vi "Text control 2 v6.6.vi"() -> ()   [LabVIEW 2016]
panel:
  in  "Tab Control":enum32{"Main", "Other parameters"}(tab)
  in  "Plot sample extrema vs time":bool
  out "Line running":i32
  out "Total lines":i32
  out "Path":path=path "C:/users/rlp38/09Apr2009LTtesting/test2.txt"
  out "I vs Vg":cluster{"Y data in":dbl[], "X data in":dbl[]}[](graph)
  out "Is max":dbl format="%.2e"
  out "Id max":dbl format="%.2e"
  out "Ig max":dbl format="%.2e"
  out "Imax vs time":cluster{"Y data in":dbl[], "X data in":dbl[]}[](graph)
  out "Imin vs time":cluster{"Y data in":dbl[], "X data in":dbl[]}[](graph)
  out "I vs Vd":cluster{"Y data in":dbl[], "X data in":dbl[]}[](graph)
  in  "Script":string="#pulsedstressV d 0.03 20 0 0.5 0.0827 5\n#\n#itime m\n#gaterangemode a\n#drainrangemode a\n#pulsed on 0.05 0 0.02\n#transfer d -10 40 1 5 40 35\n#transfer d -10 40 1 5 40 35\n#transfer d -10 40 1 5 40 35\n#output d 0 40 20 0 40 1\n#\n#\n#sample 1 0.008 221 6 0.003\n#samplei 400e-6 200 6 0.002 0.1\n#vsu2pulse -10 4\n#\n#stressV 0.016 0.03 2e-4 0.1e-3 11\n#stressI 220e-7 0.08 15\n#transfer s -1 1 0.5 -0.005 0.005 0.005\n#output s 0 0 0 -0.008 0.008 0.002"
  out "Command running:":string
  out "Serial port data":string
  out "Elapsed Time":dbl caption="Elapsed Time (s)"
  in  "Time Units":u16(ring)=1 items=["Seconds", "Minutes", "Hours"]
  in  "Time Offset":dbl caption="Set Start Time (s)"
  in  "Reset":bool
  in  "Auto Reset":bool
  in  "integration time":u32(slide) max=2 step=1 scale=0.0..2.0
  out "Is on":dbl format="%.2e"
  out "Id on":dbl format="%.2e"
  out "Ig on":dbl format="%.2e"
  out "Ion vs time":cluster{"Y data in":dbl[], "X data in":dbl[]}[](graph)
  out "Ioff vs time":cluster{"Y data in":dbl[], "X data in":dbl[]}[](graph)
  out "Ig min":dbl format="%.2e"
  out "Id min":dbl format="%.2e"
  out "Is min":dbl format="%.2e"
  out "Is off":dbl format="%.2e"
  out "Id off":dbl format="%.2e"
  out "Ig off":dbl format="%.2e"
  in  "Integration time (long)":dbl=0.32 min=0.04 max=2.0 step=0.02 format="%.2f"
  in  "Integration time (short)":dbl=0.0019 min=8e-05 max=0.0019 step=8e-05 format="%^.0e"
  in  "Drain: Compliance":dbl=0.001 format="%.8f"
  in  "Gate: Compliance":dbl=0.001 format="%.8f"
  in  "Interrupt scan":bool
  in  "Interrupt program":bool
  in  "Plot output curve extrema vs time":bool
  in  "Plot transfer curve extrema vs time":bool
  out "I vs time (Bias Stress)":cluster{"Y data in":dbl[], "X data in":dbl[]}[](graph)
  in  "Gate Range\nmode":u16(ring) items=["Auto", "Limited", "Fixed"]
  in  "Gate Range":u8(slide)=6 max=11 scale=0.0..11.0
  in  "Source/Drain\nRange mode":u16(ring) items=["Auto", "Limited", "Fixed"]
  in  "Source/Drain Range":u8(slide)=6 max=11 scale=0.0..11.0
  in  "Panel Controls":T1={"Emergency Stop"=refnum, "TransGraph Max"=1e-05, "Text/Graph (text=false)"=TRUE} {"TransGraph Max" format="%.2e"}
  in  "Panel Controls 2":T2={"Emergency Stop"=refnum, "TransGraph Max"=1e-05, "Text/Graph (text=false)"=TRUE, "TransGraph Min"=1e-11} {"TransGraph Min" format="%.2e"; "TransGraph Max" format="%.2e"}
  out "error out":errorcluster
  in  "Delay before read (ms)":u32=1000
  in  "byte count":u32=64
  in  "Serial End Mode for Reads":u16(ring)=2 items=["None", "LastBit", "TermChar"]
  in  "Timeout (ms)":u32=10000
  in  "Enable Termination\nChar (T)":bool=TRUE
  in  "Termination char\n(0xA = '\\n' = LF)\n(0xD = '\\r' = CR)":u8=13 format="%.0x"
  in  "flow control":u16(ring) items=["None"=0, "XON/XOFF"=1, "RTS/CTS"=2, "DTR/DSR"=4]
  in  "stop bits":u16(ring)=10 items=["1.0"=10, "1.5"=15, "2.0"=20]
  in  "parity":u16(ring) items=["None", "Odd", "Even", "Mark", "Space"]
  in  "data bits":u16=8 min=5 max=8 step=1
  in  "VISA resource name":refnum<visa-resource-name>="COM6"
  in  "baud rate":u32=9600
  out "Timings Indicator":T3
  in  "Timings (overwritten by the Front Panel)":T4={"integration time"=0, "Short/Long integration time"=0.00064, "hold time (sec)"=0.0, "delay time (sec)"=0.0, "Step Time (0 disables)"=0.0, "sweep method"=0, "Pulse period"=0.005, "Base voltage"=0.0, "Pulse width"=0.0005} {"Pulse width" min=0.0005 max=0.1 step=0.0001 format="%.4f"; "Base voltage" format="%^.4e"; "Pulse period" min=0.005 max=1.0 step=0.0001 format="%.4f"; "sweep method" items=["Continuous", "Pulsed"]; "Step Time (0 disables)" format="%.2f"; "delay time (sec)" format="%.4f"; "hold time (sec)" format="%.4f"; "Short/Long integration time" format="%^.0e"; "integration time" scale=0.0..2.0}
  in  "SMU4":cluster{"on/off":bool, "Voltage":dbl} {"Voltage" min=-100.0 max=100.0 format="%.2f"}
  in  "Full Reset":bool
  in  "Standby":T5
  out "SMU4 Indicator":cluster{"on/off":bool, "Voltage":dbl} {"Voltage" min=-100.0 max=100.0 format="%.2f"}
  in  "Gate":T6={"Gate Start"=0.0, "Gate Stop"=2.0, "Gate Step (linear only)"=1.0, "Gate Compliance"=0.0001, "Gate PComp"=0.0, "Range mode"=0, "Range"=6} {"Range" max=11 scale=0.0..11.0; "Range mode" items=["Auto", "Limited", "Fixed"]; "Gate PComp" format="%^.2e"; "Gate Compliance" format="%^.2e"; "Gate Step (linear only)" format="%^.4e"; "Gate Stop" format="%^.4e"; "Gate Start" format="%^.4e"}
  in  "Drain 2":T7={"Drain Start"=0.0, "Drain Stop"=2.0, "Drain Compliance"=0.0001, "Drain Step"=1.0, "Drain PComp"=0.0, "Range mode"=0, "Range"=6} {"Range" max=11 scale=0.0..11.0; "Range mode" items=["Auto", "Limited", "Fixed"]; "Drain PComp" format="%^.2e"; "Drain Step" format="%^.4e"; "Drain Compliance" format="%^.2e"; "Drain Stop" format="%^.4e"; "Drain Start" format="%^.4e"}
  # "Time"
  # "Syntax:\nitime [s|m|l] time(sec): [s|m|l] determines the integration time setting (small|medium|long) and time sets the value.\nNOTE: The value of the integration time has to be within the range allowed by its category (s|m|l), otherwise, the closest value will be used. (e.g. if the category is set to short but the time value is very long, the actual value used will be the maximum short integration time.\nIntegration times:\n    Short: Default: 640 us. Range: 8E-5 - 1.92E-3 seconds.\n    Medium: Fixed at 1 NPL cycle (0.02 seconds).\n    Long: Default: 16 NPL cycles (0.32 seconds). Range: 2-100 NPL cycles (0.04 seconds - 2 seconds).\ngaterangemode [a|l|f]\ndrainrangemode [a|l|f]\npulsed [on|off] PulsePeriod(sec) PulseBaseVoltage PulseONWidth(sec)\nstandby [on l off]\nwait NumMilliseconds\nwait-min NumMinutes\n# texthere = comment\nSMU4 [ON|OFF] Voltage\ntransfer [s|d] VgStart VgStop VgStep VdStart VdStop VdStep\noutput [s|d] VgStart VgStop VgStep VdStart VdStop VdStep\nsample Vg Vd NumSamples Time(s) SampleInterval(s)\nsamplei Idg NumSamples Time(s) SampleInterval(s) VDGcompliance\n100 samples is approximately 13 seconds with medium integration\n# if in doubt use SampleInterval(s) = 0.004\n    NOTE: When doing bias stress measurements, set the Time Units to \"Seconds\", as the \"sample\" command has been configured to give the output to seconds.\nstressV VG VD IGcompliance IDcompliance Duration(sec)\nstressI IDG VDGcompliance Duration(sec)\nvsu2pulse Bias Duration(s)\npulsedstressV [s|d] VEstop VgON VgOFF Period(s) PulseONwidth(s) Vd\nsample-fpp Vg Vd NumSamples Time\nresample-fpp Vg Vd\ntransfer-fpp [s|d] VgStart VgStop VgStep VdStart VdStop VdStep\noutput-fpp [s|d] VgStart VgStop VgStep VdStart VdStop VdStep\nserial SerialPortCommand"
  # "1\n2\n3\n4\n5\n6\n7\n8\n9\n10\n11\n12\n13\n14\n15\n16\n17\n18\n19\n20"
  # "Serial port settings"
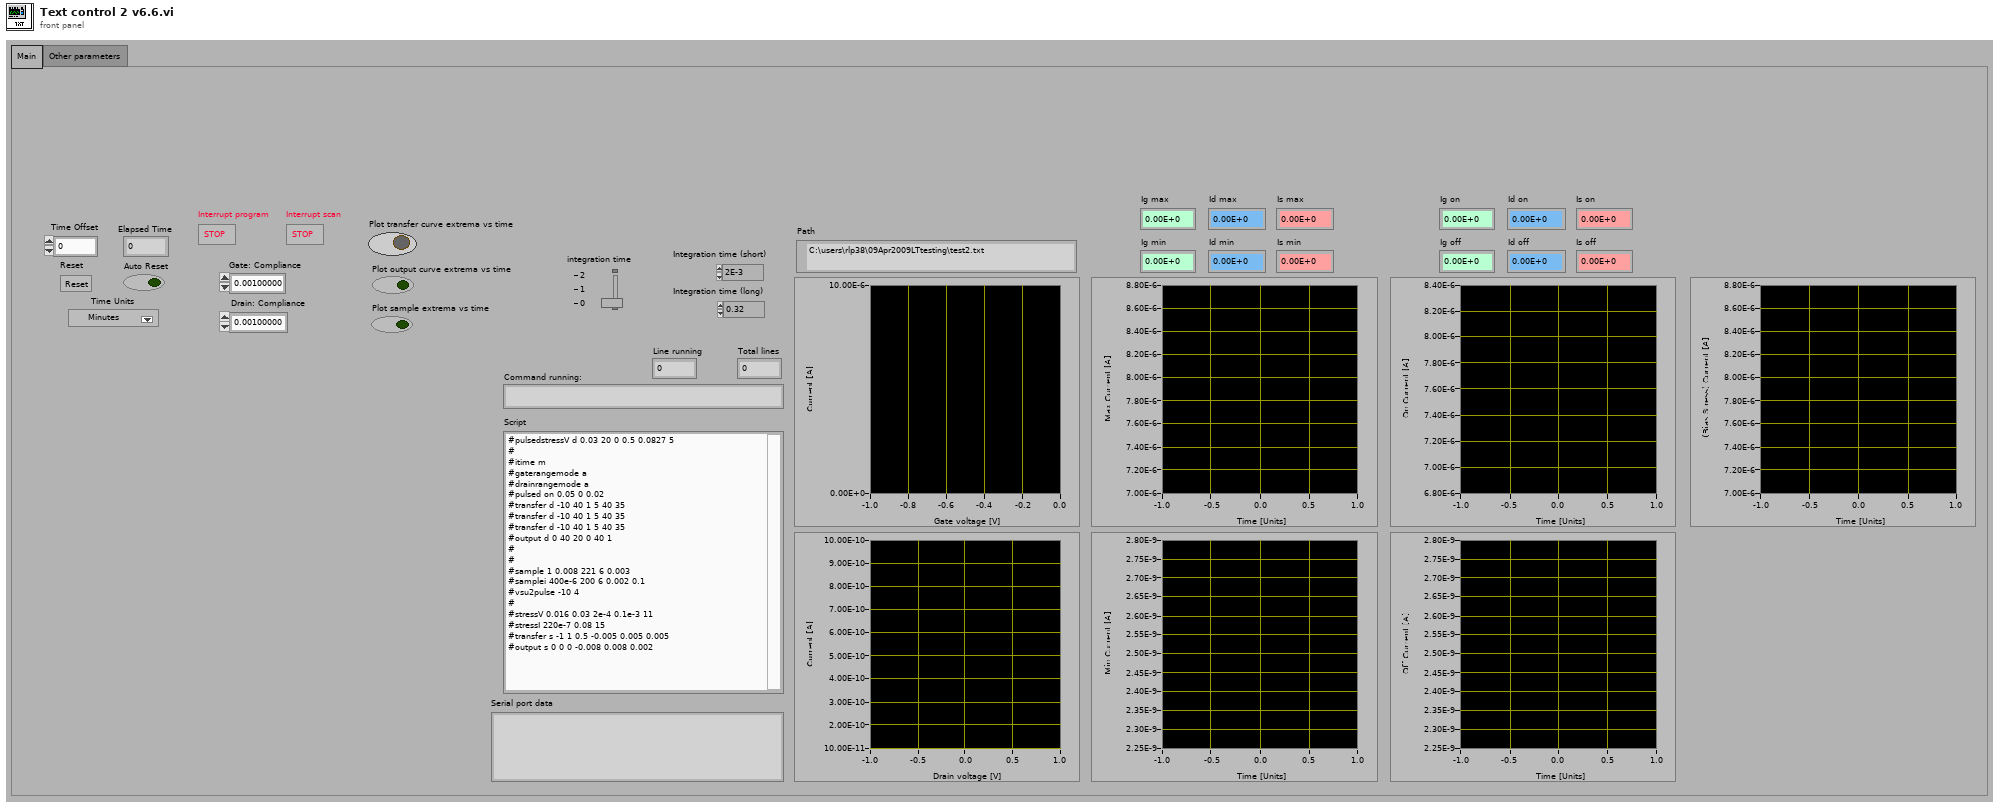
[diagram p1: front panel]
types:
  T1 = cluster{"Emergency Stop":refnum<vi>, "TransGraph Max":dbl, "Text/Graph (text=false)":bool}
  T2 = cluster{"Emergency Stop":refnum<vi>, "TransGraph Max":dbl, "Text/Graph (text=false)":bool, "TransGraph Min":dbl}
  T3 = cluster{"integration time (0:s, 1:m, 2:l)":u32, "Short/Long integration time":dbl, "hold time (sec)":dbl, "delay time (sec)":dbl, "Step Time (0 disables)":dbl, "sweep method":u16, "Pulse period":dbl, "Base voltage":dbl, "Pulse width":dbl}
  T4 = cluster{"integration time":u32, "Short/Long integration time":dbl, "hold time (sec)":dbl, "delay time (sec)":dbl, "Step Time (0 disables)":dbl, "sweep method":u16, "Pulse period":dbl, "Base voltage":dbl, "Pulse width":dbl}
  T5 = cluster{"Gate Standby":bool, "Drain Standby":bool}
  T6 = cluster{"Gate Start":dbl, "Gate Stop":dbl, "Gate Step (linear only)":dbl, "Gate Compliance":dbl, "Gate PComp":dbl, "Range mode":u16, "Range":u8}
  T7 = cluster{"Drain Start":dbl, "Drain Stop":dbl, "Drain Compliance":dbl, "Drain Step":dbl, "Drain PComp":dbl, "Range mode":u16, "Range":u8}
  T8 = enum16{"open", "replace", "create", "open or create", "replace or create", "replace or create with confirmation"}
  T9 = cluster{"V2 Start":dbl, "V2 Step":dbl, "Number of points":i32}
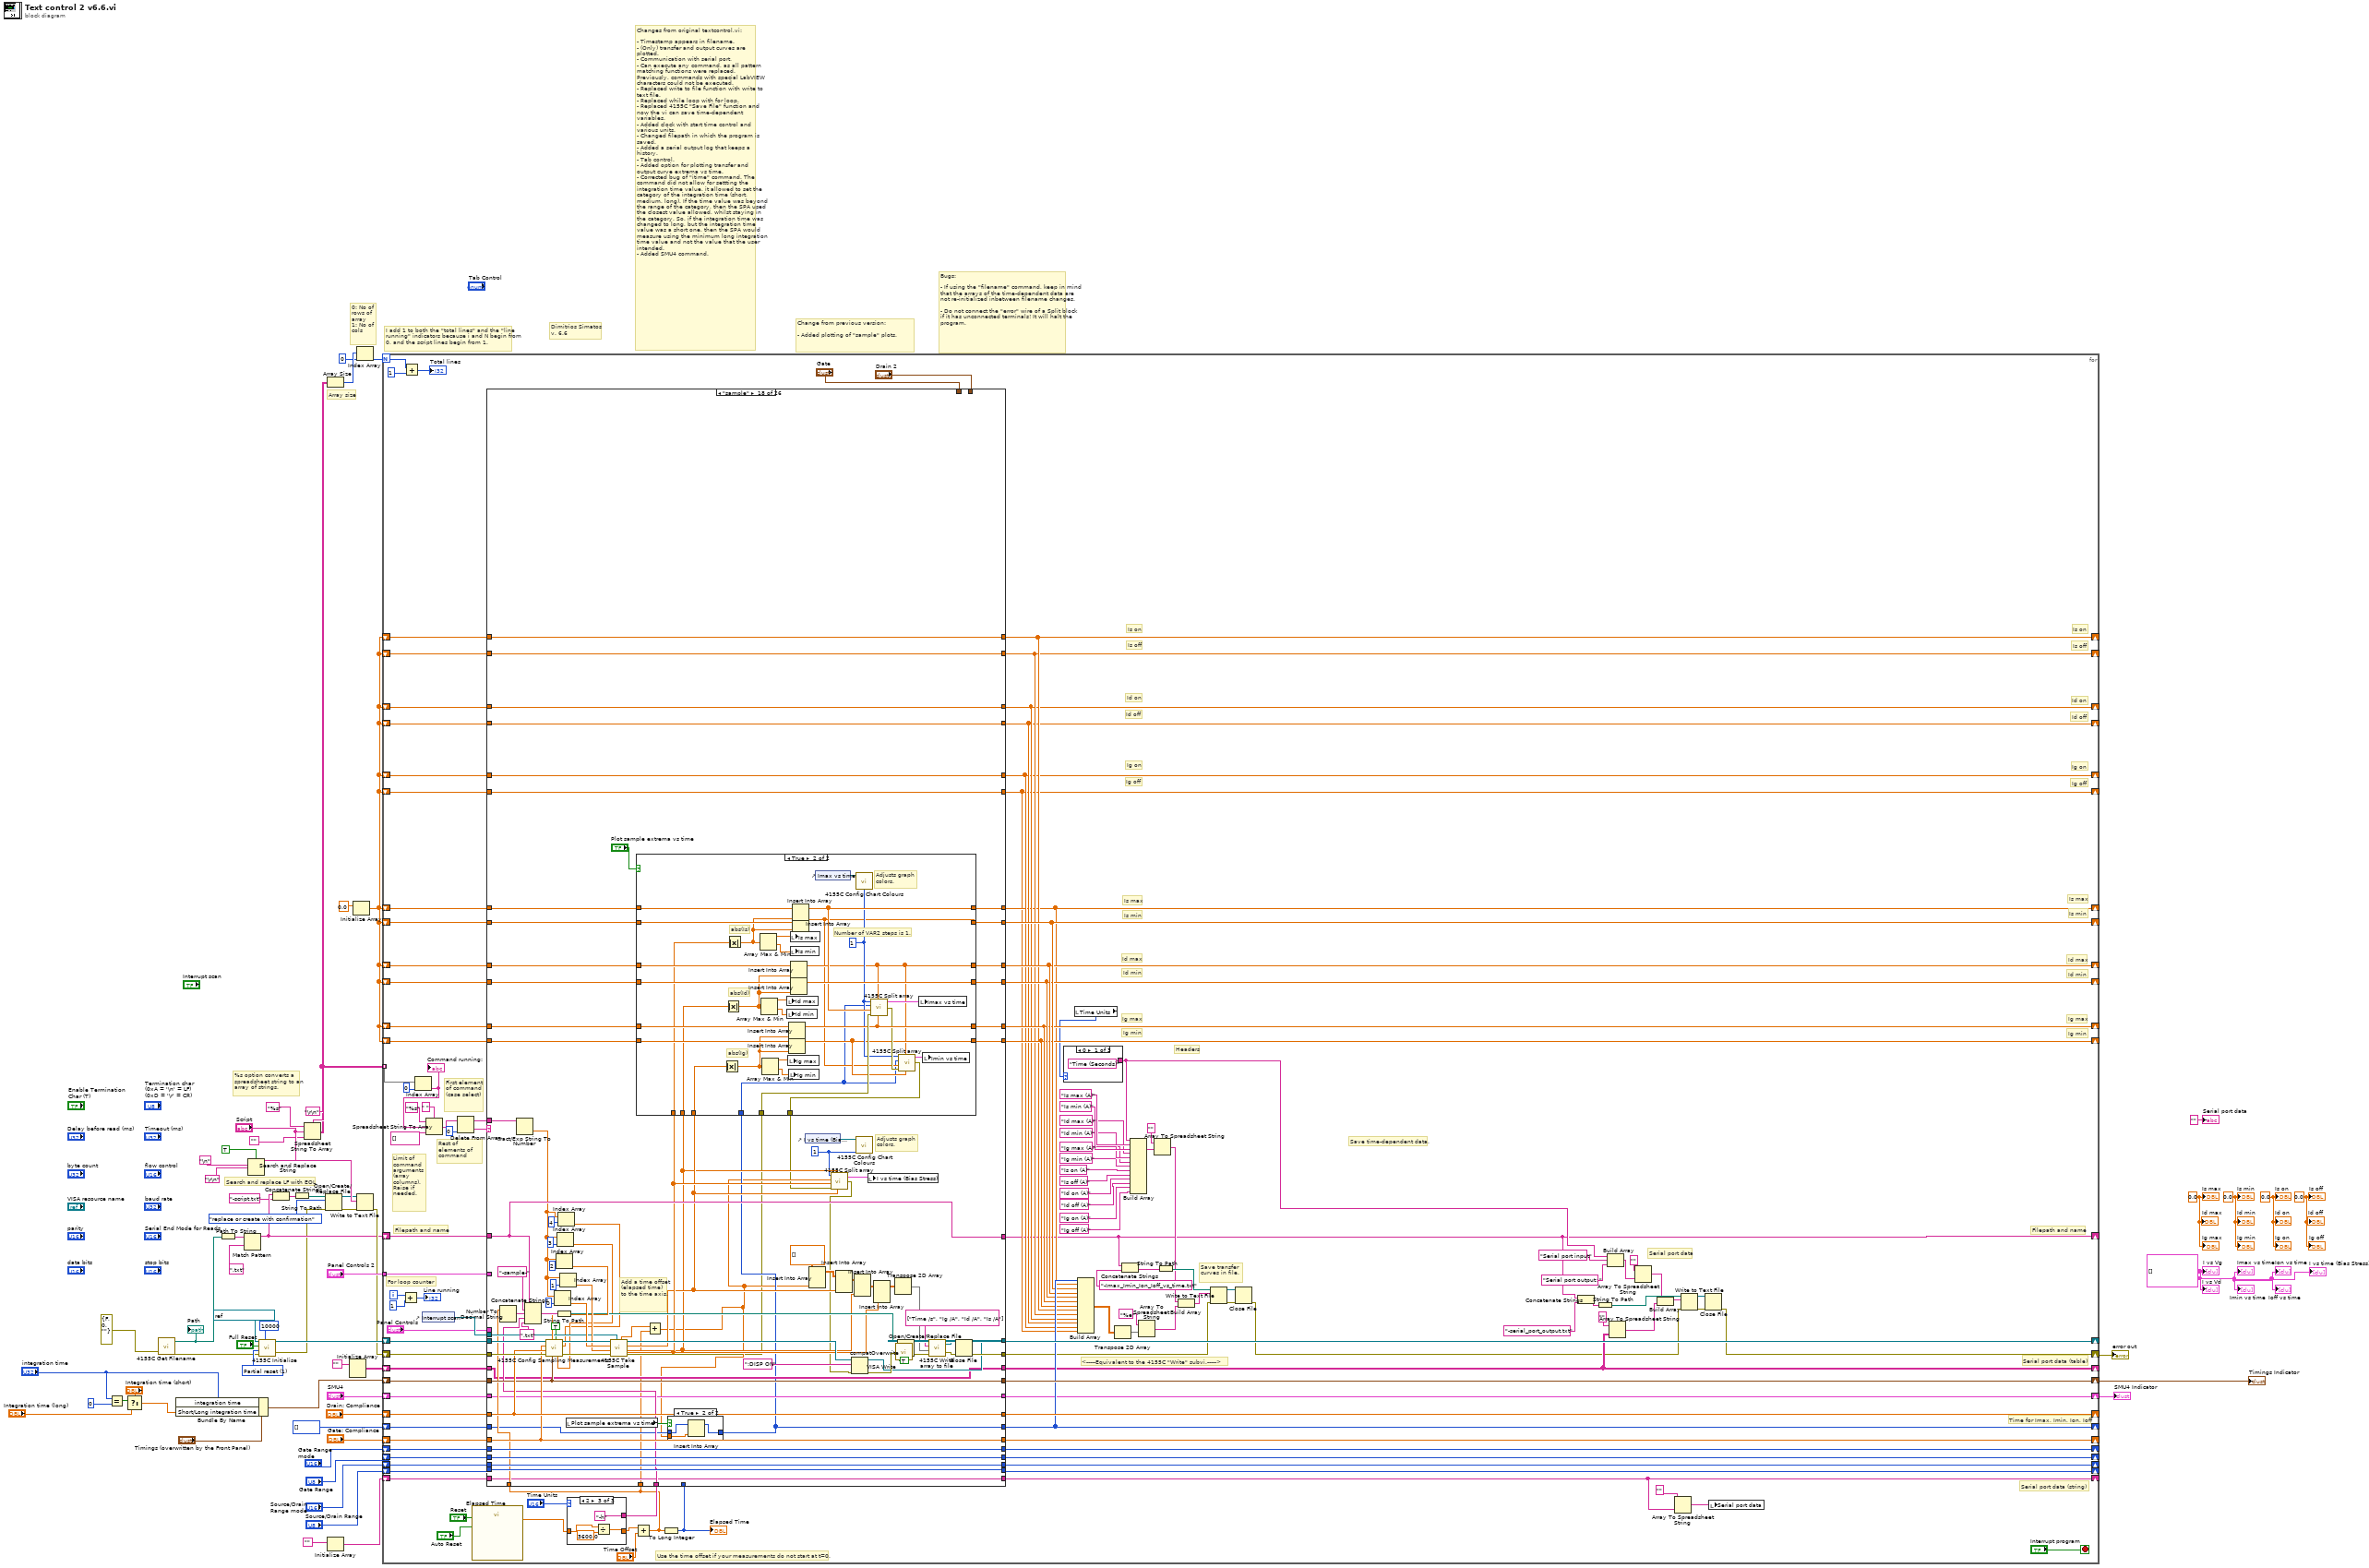
[diagram p0: block diagram]
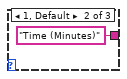
[diagram p2: hidden frame]
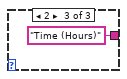
[diagram p3: hidden frame]
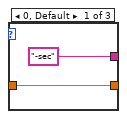
[diagram p4: hidden frame]
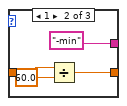
[diagram p5: hidden frame]
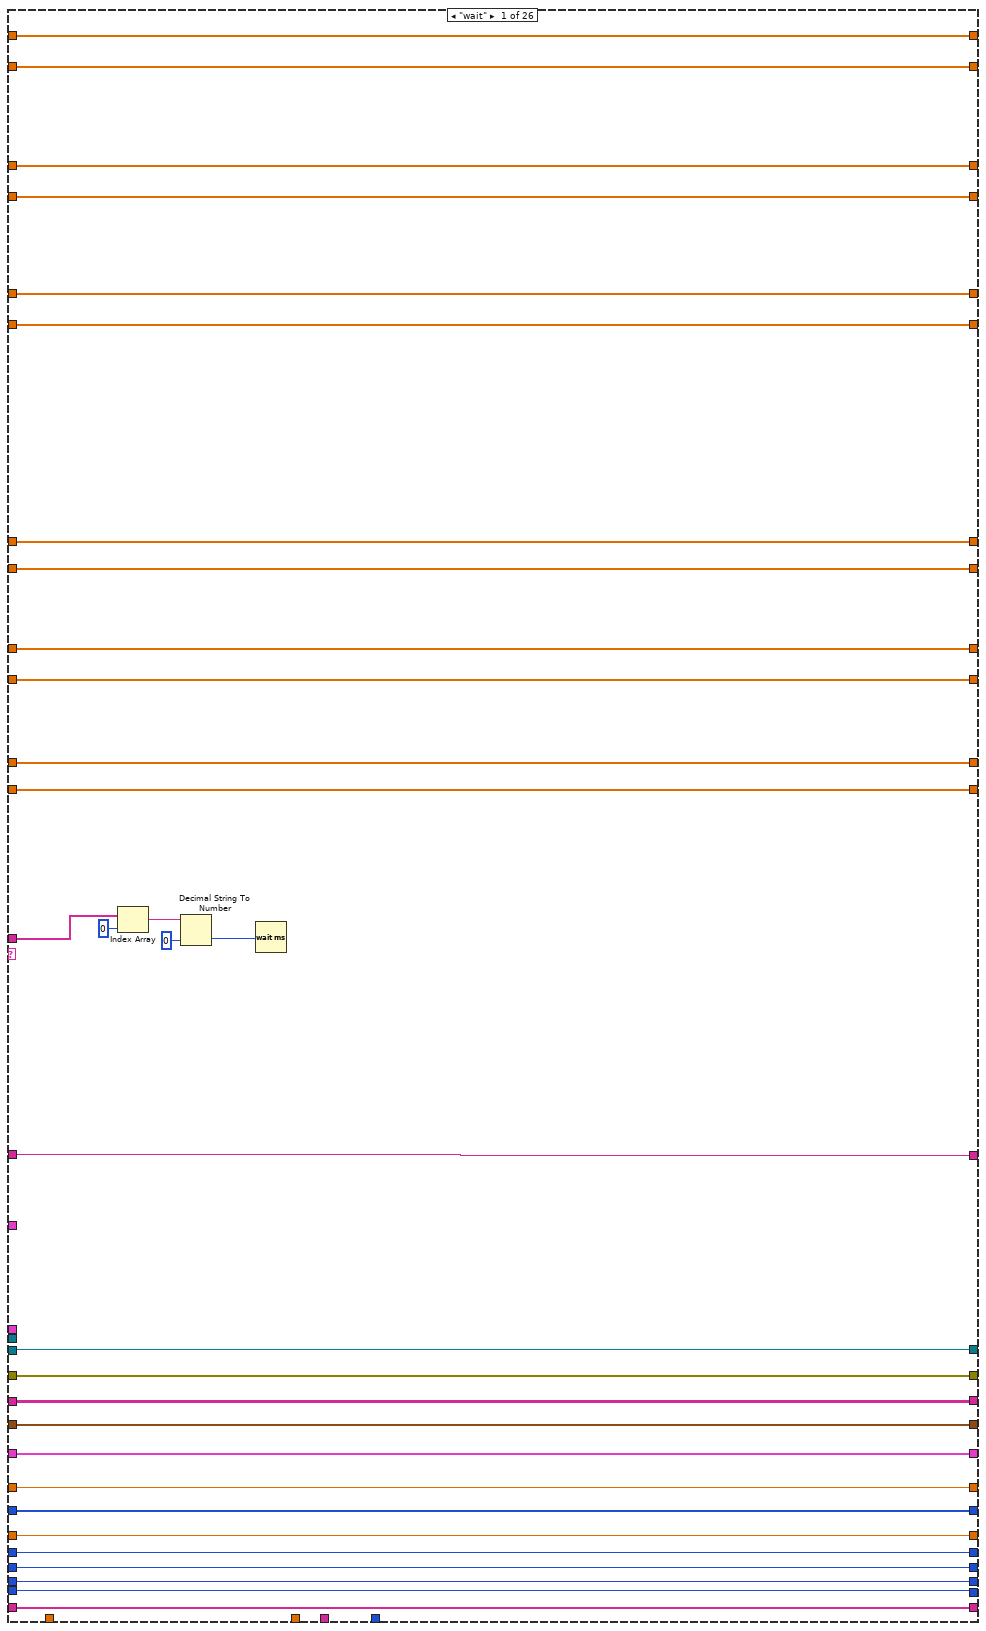
[diagram p6: hidden frame]
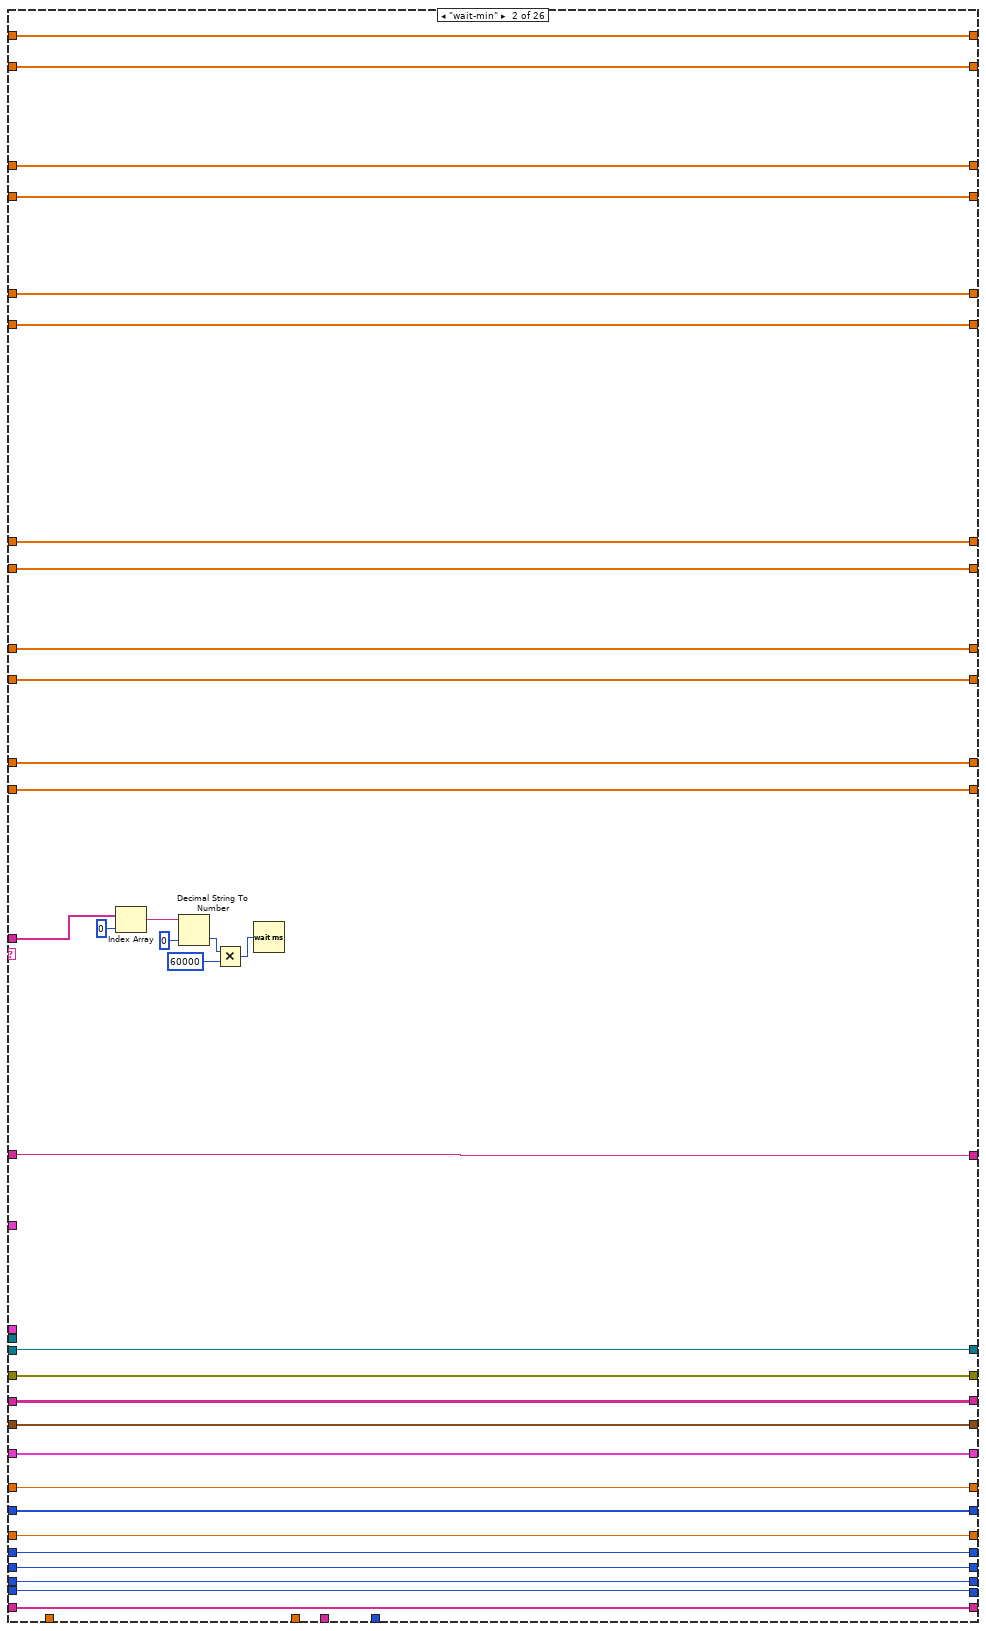
[diagram p7: hidden frame]
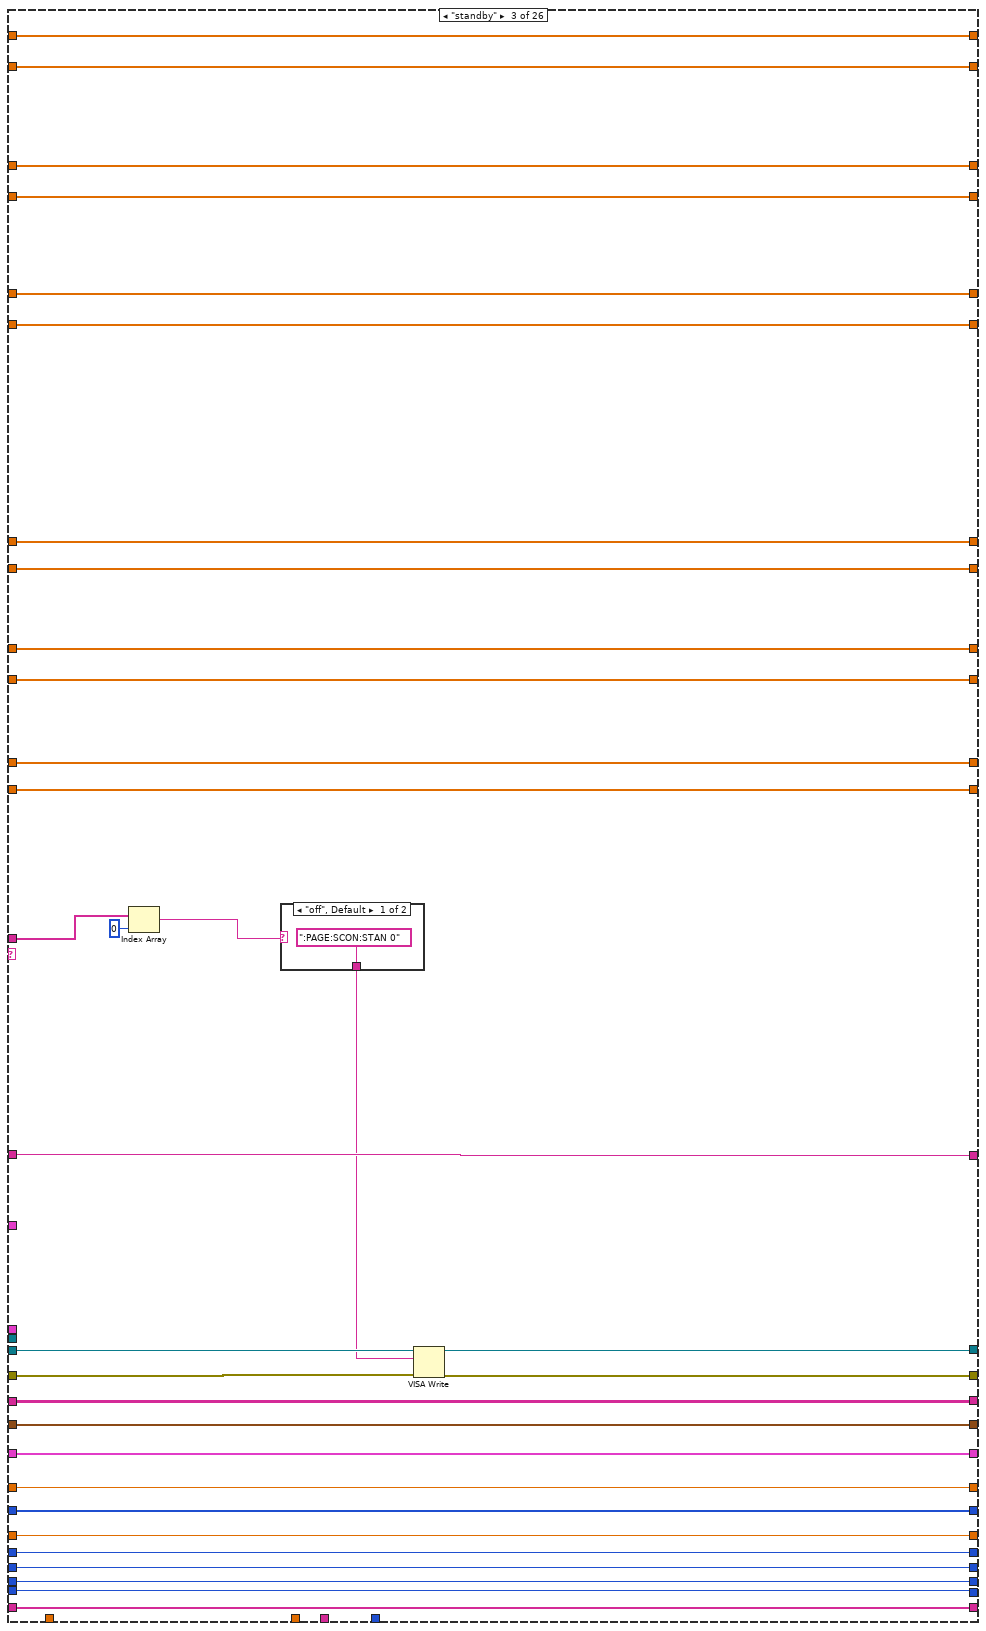
[diagram p8: hidden frame]
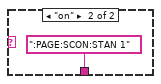
[diagram p9: hidden frame]
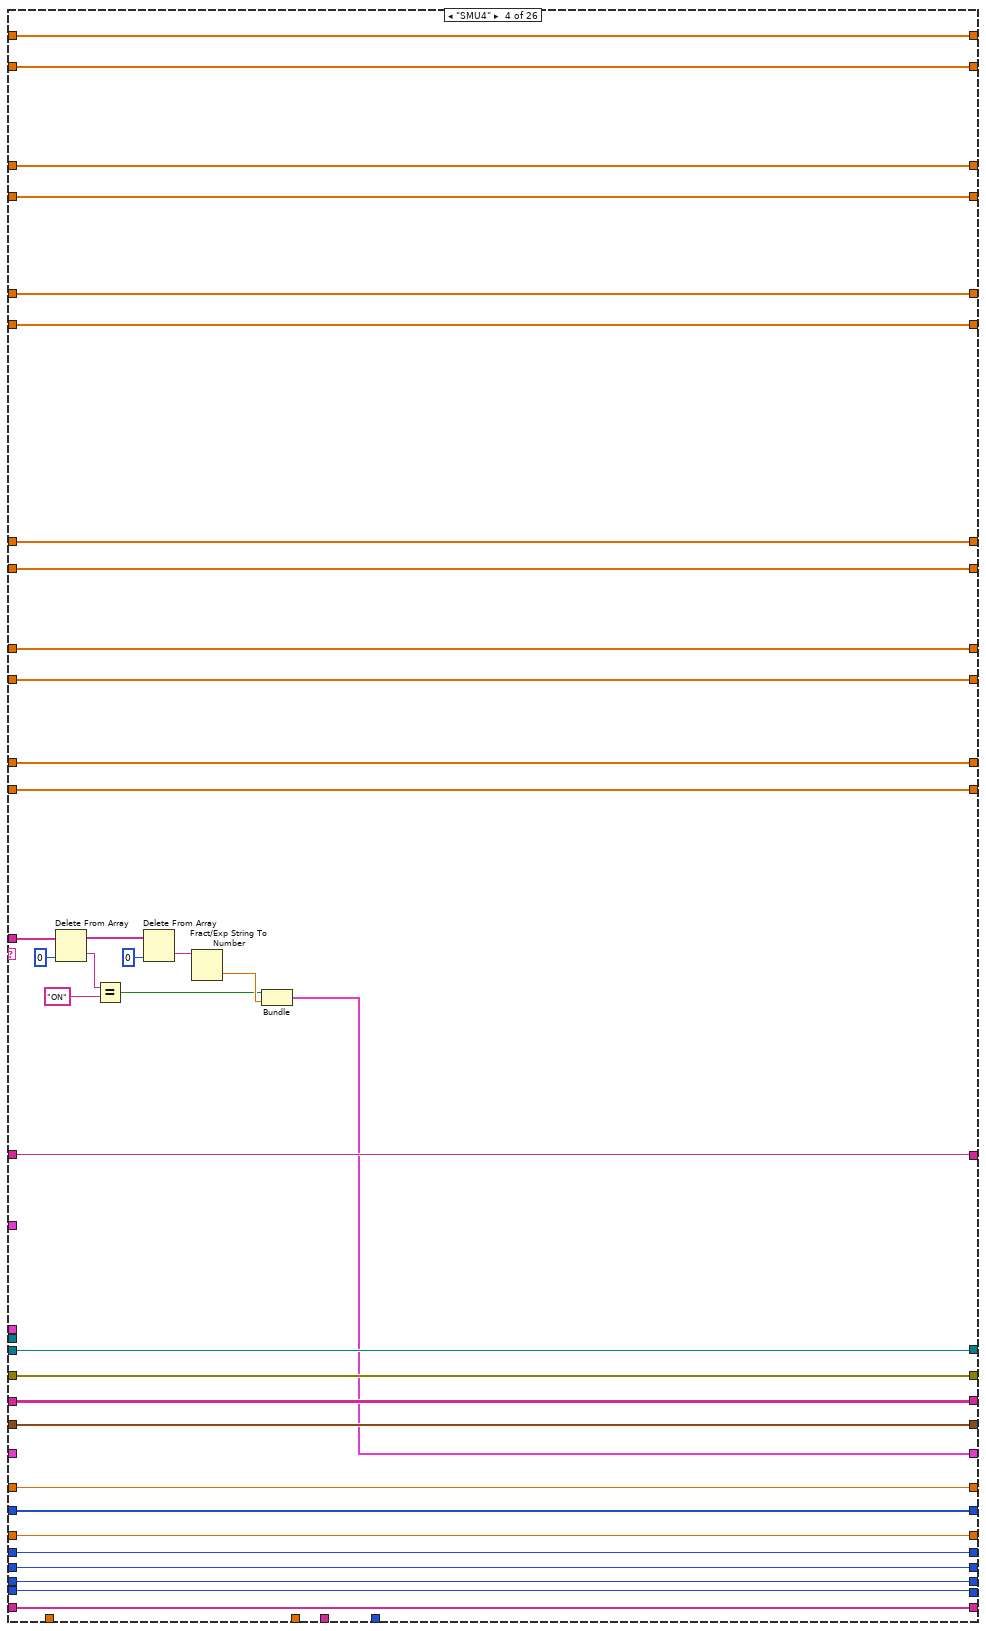
[diagram p10: hidden frame]
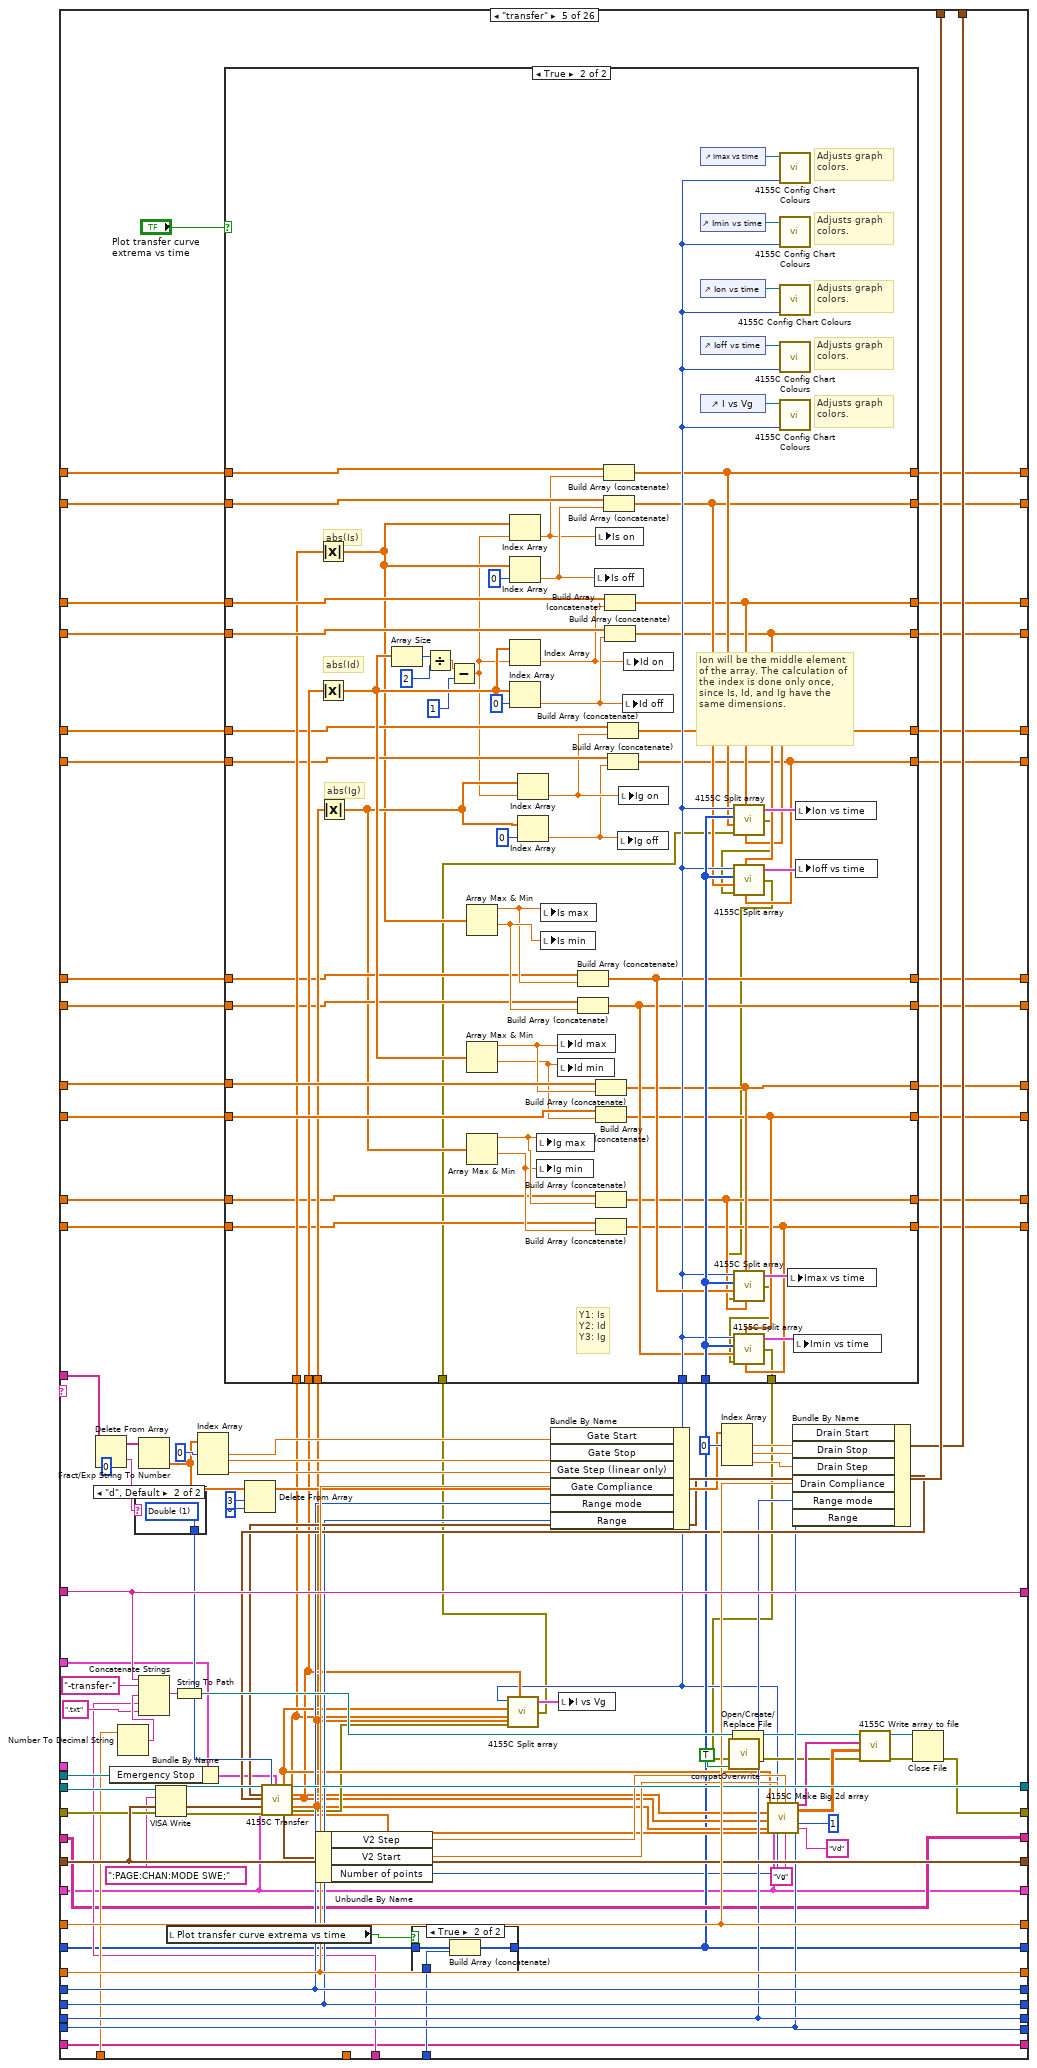
[diagram p11: hidden frame]
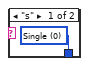
[diagram p14: hidden frame]
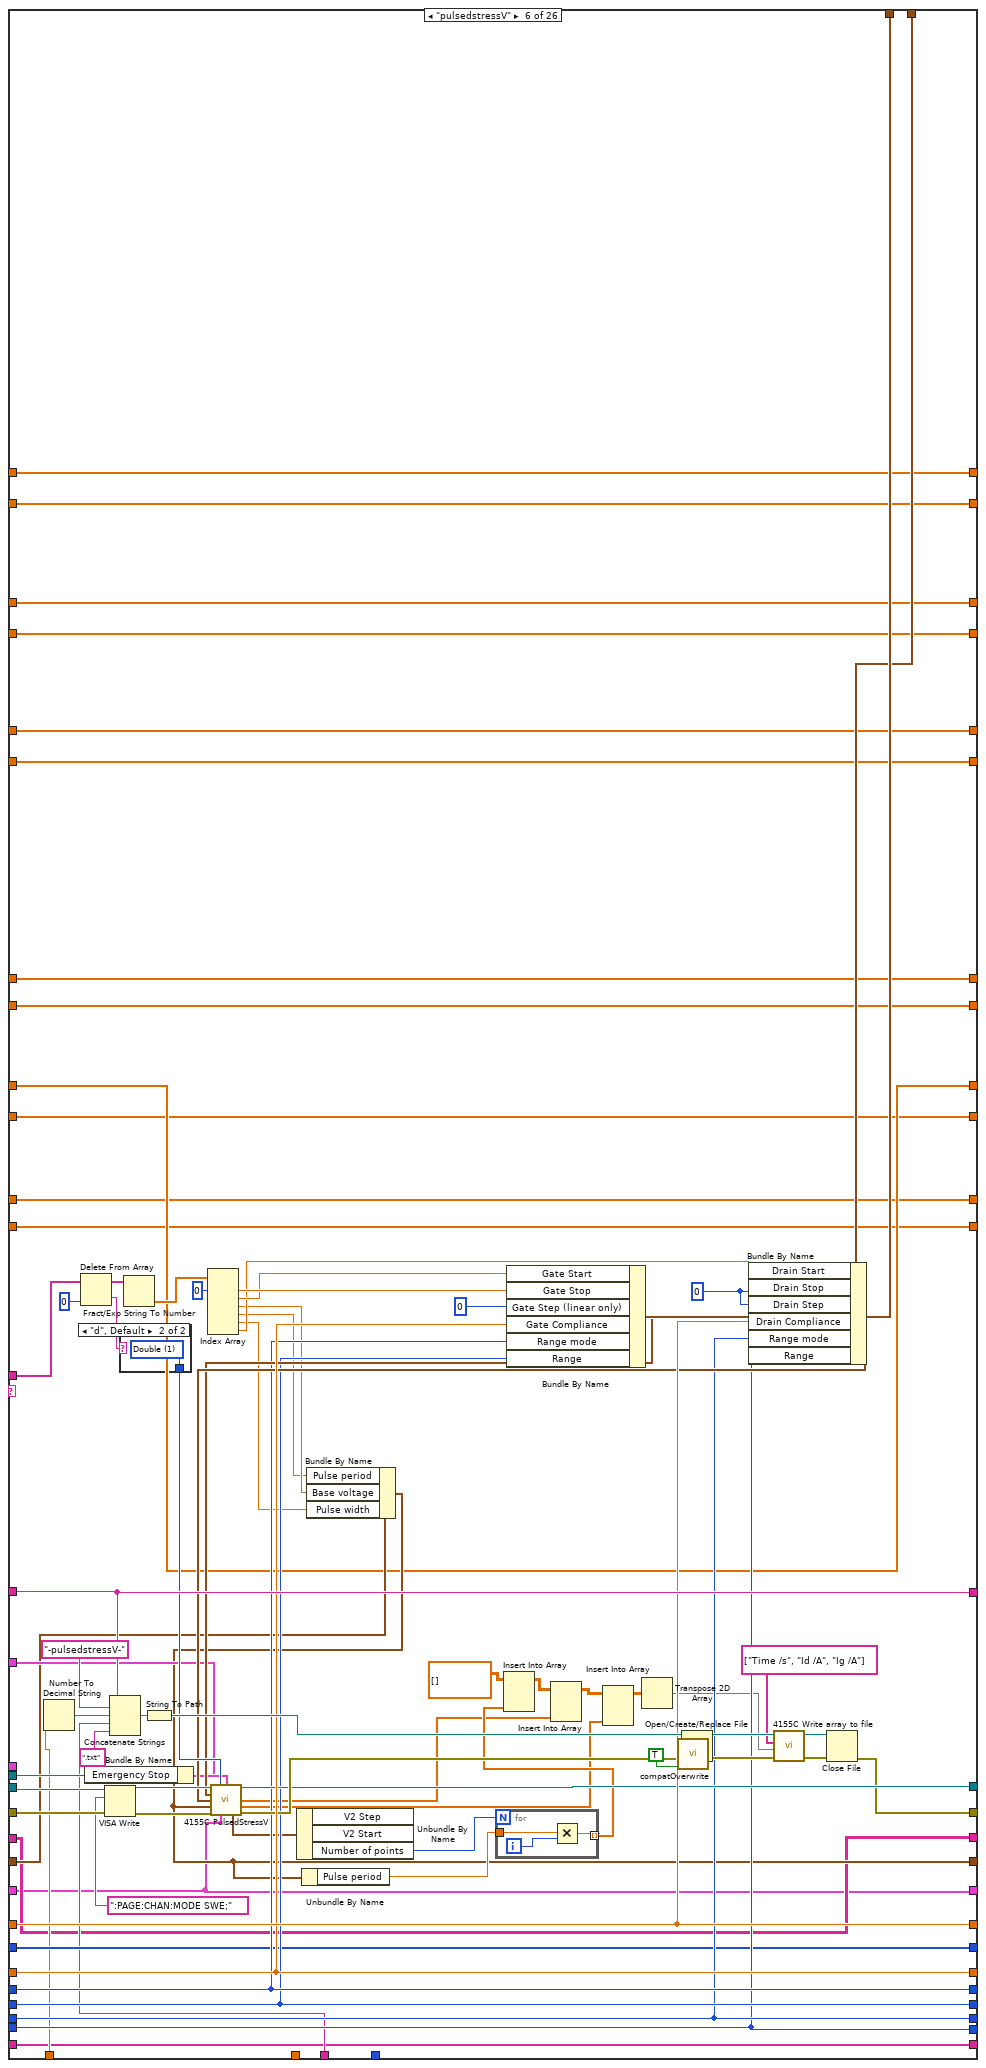
[diagram p15: hidden frame]
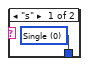
[diagram p16: hidden frame]
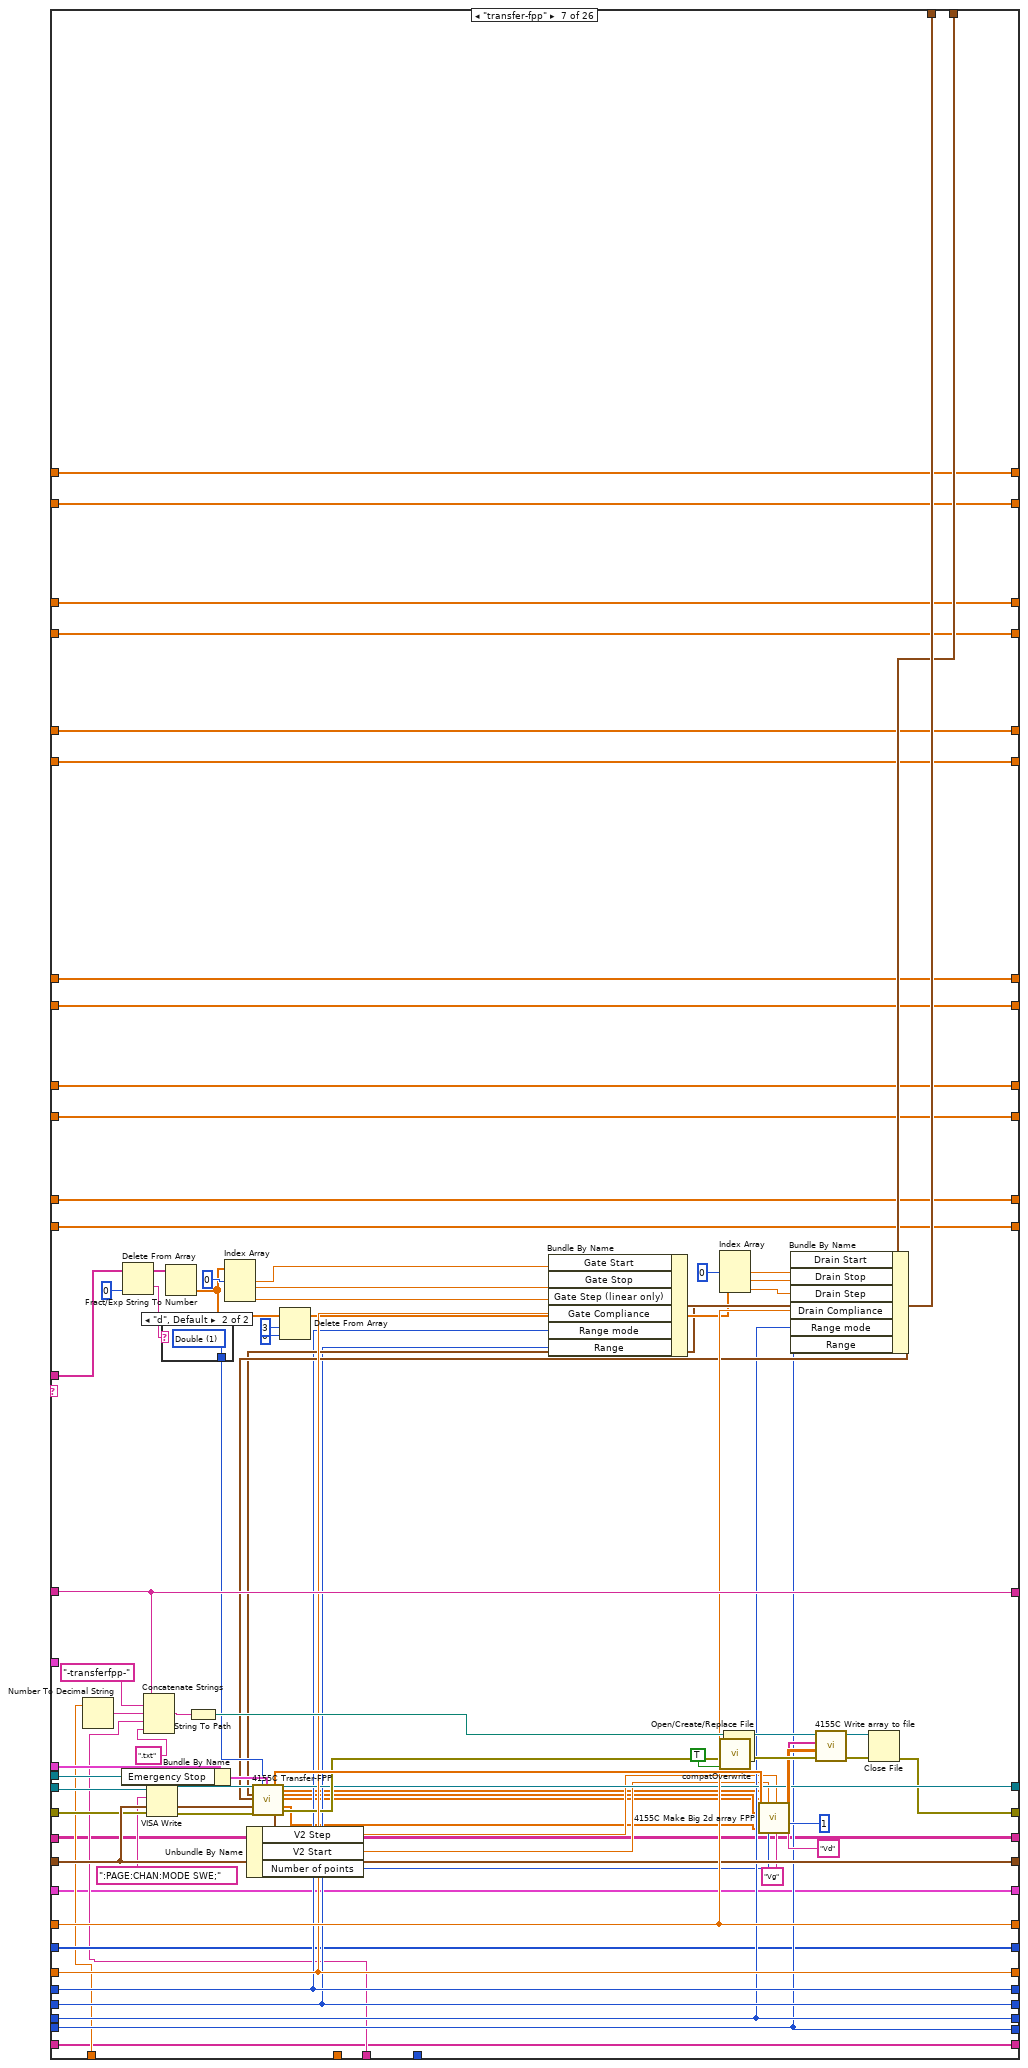
[diagram p17: hidden frame]
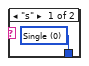
[diagram p18: hidden frame]
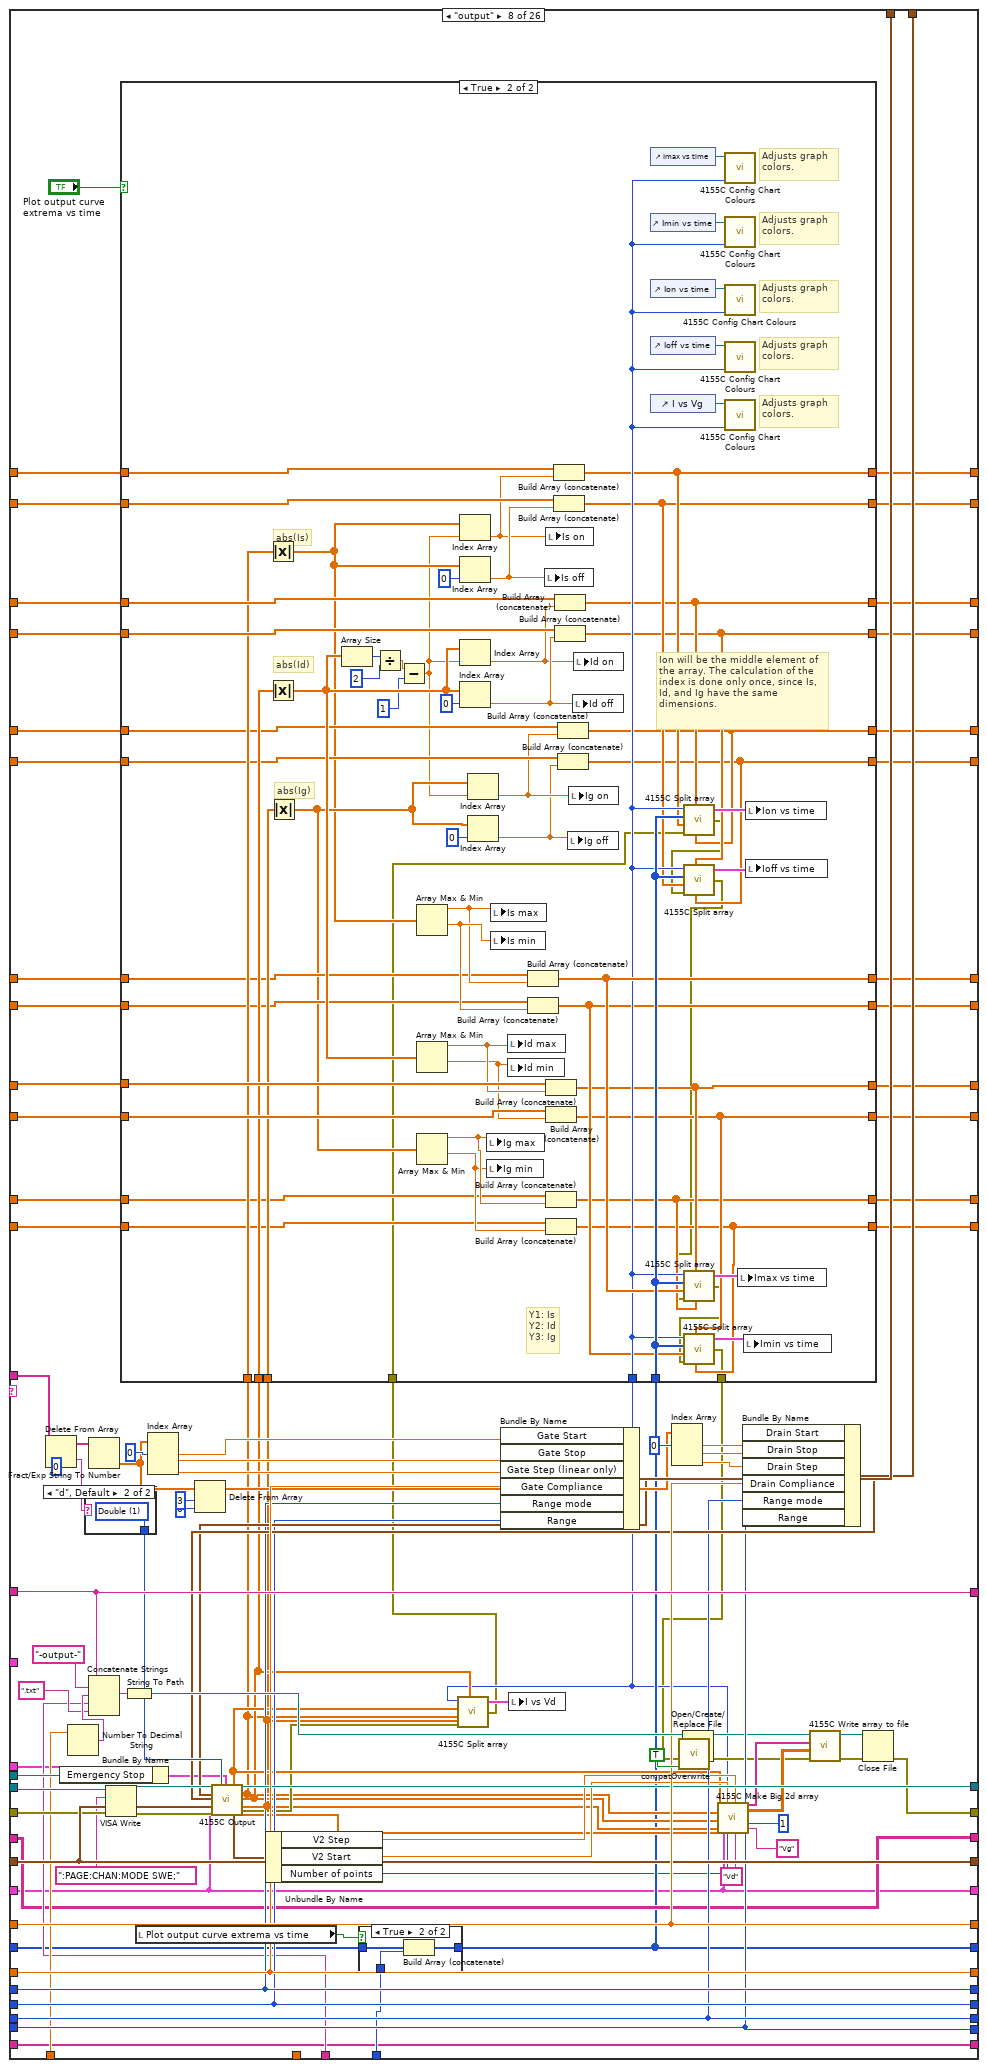
[diagram p19: hidden frame]
diagram:
  w1 = cluster{"Y data in":dbl[], "X data in":dbl[]}[] [] ("I vs Vg")
  w9 = 0.0 ("Is off")
  w10 = 0.0 ("Is on")
  w11 = 0.0 ("Is min")
  w12 = 0.0 ("Is max")
  w58 = u16 1 items=["Reset All", "Partial reset"] ("Type of reset")
  # "Change from previous version:\n\n- Added plotting of \"sample\" plots."
  # "I add 1 to both the \"total lines\" and the \"line running\" indicators because i and N begin from 0, and the script lines begin from 1."
  # "Bugs:\n\n- If using the \"filename\" command, keep in mind that the arrays of the time-dependent data are not re-initialized inbetween filename changes. \n\n- Do not connect the \"error\" wire of a Split block if it has unconnected terminals! It will halt the program."
  # "Array size"
  # "%s option converts a spreadsheet string to an array of strings."
  # "0: No of rows of array\n1: No of cols"
  # "Dimitrios Simatos\nv. 6.6"
  # "Changes from original textcontrol.vi:\n\n- Timestamp appears in filename.\n- (Only) transfer and output curves are plotted.\n- Communication with serial port.\n- Can execute any command, as all pattern matching functions were replaced. Previously, commands with special LabVIEW characters could not be executed.\n- Replaced write to file function with write to text file.\n- Replaced while loop with for loop.\n- Replaced 4155C \"Save File\" function and now the vi can save time-dependent variables.\n- Added clock with start time control and various units.\n- Changed filepath in which the program is saved.\n- Added a serial output log that keeps a history.\n- Tab control.\n- Added option for plotting transfer and output curve extrema vs time.\n- Corrected bug of \"itime\" command. The command did not allow for settting the integration time value, it allowed to set the category of the integration time (short, medium, long). If the time value was beyond the range of the category, then the SPA used the closest value allowed, whilst staying in the category. So, if the integration time was changed to long, but the integration time value was a short one, then the SPA would measure using the minimum long integration time value and not the value that the user intended.\n- Added SMU4 command."
  # "Search and replace LF with EOL"
  n1 = Equal?(x="integration time", y=u32 0) -> (x = y?=w59:bool)
  n2 = Select(t="Integration time (short)", s=w59, f="Integration time (long)") -> (s? t:f=w17:dbl)
  n3 = call "4155C Get Filename.vi"("error in (no error)"=errorcluster {"status"=FALSE, "code"=0, "source"=""}) -> ("error out"=w53:errorcluster, "path"=w28:path)  [unwired: 2 in, 1 out]
  "Path" <- w28
  n4 = Bundle By Name(cluster="Timings (overwritten by the Front Panel)", "integration time"="integration time", "Short/Long integration time"=w17) -> (w51:T4)
  n5 = Path To String(path=w28) -> (string=w29:string)
  n6 = Match Pattern(string=w29, regular expression=".txt") -> (before substring=w15:string)  [unwired: 1 in, 3 out]
  n7 = Search and Replace String(replace all?=TRUE ("replace all? (F)"), input string="Script", search string="\n", replace string="\r\n") -> (result string=w41:string)  [unwired: 4 in, 3 out]
  n8 = call "4155C Initialise.vi"("VISA resource name in"=refnum<visa-resource-name> "GPIB0::14::INSTR", "Reset"="Full Reset", "Type of reset"=w58, "error in (no error)"=w53, "VISA Timeout Value"=u32 10000) -> ("VISA Resource Name out"=w52:refnum<visa-resource-name>, "error out"=w7:errorcluster)
  n9 = Concatenate Strings(w15, "-script.txt" ("string")) -> (w16:string)
  n10 = String To Path(string=w16) -> (path=w5:path)
  n11 = Spreadsheet String To Array(delimiter (Tab)="\r\n", format string="%s", spreadsheet string="Script", array type (2D Dbl)="") -> (array=w32:string[][])
  n12 = Open/Create/Replace File(file path (use dialog)=w5, error in=w7, operation (0:open)=T8."replace or create with confirmation") -> (refnum out=w4:refnum<file>, error out=w6:errorcluster)  [unwired: 3 in, 1 out]
  n13 = Array Size(array=w32) -> (size(s)=w36:i32[])
  n14 = Initialize Array("") -> (w21:string[])  [unwired: 1 in]
  n15 = Initialize Array("") -> (w19:string[][])  [unwired: 2 in]
  n16 = Initialize Array(0.0 ("element")) -> (w23:dbl[])  [unwired: 1 in]
  n17 = Index Array(array=w36, index=0) -> (element=w34:i32)
  n18 = Write to Text File(file (use dialog)=w4, text=w41, error in=w6) -> (error out=w25:errorcluster)  [unwired: 1 in, 2 out]
  n19 = for {
    N: w34 -> [w133]
    shift-left: "Source/Drain Range" -> [w173]
    shift-right: [w169] -> _
    shift-left: "Source/Drain\nRange mode" -> [w174]
    shift-right: [w170] -> _
    shift-left: "Gate Range" -> [w175]
    shift-right: [w171] -> _
    shift-left: "Gate Range\nmode" -> [w176]
    shift-right: [w172] -> _
    shift-left: "Gate: Compliance" -> [w185]
    shift-right: [w181] -> _
    shift-left: "Drain: Compliance" -> [w186]
    shift-right: [w182] -> _
    shift-left: w51 -> [w187]
    shift-right: [w183] -> w18
    shift-left: w25 -> [w188]
    shift-right: [w70] -> w27
    shift-left: w52 -> [w189]
    shift-right: [w184] -> _
    shift-left: w15 -> [w190]
    shift-right: [w73] -> _
    tunnel: "Panel Controls 2" -> [w167]
    shift-right: [w85] -> _
    shift-left: w23 -> [w166]
    shift-right: [w120] -> _
    shift-left: i32[] [] -> [w162]
    tunnel: w32 -> [w161] mode=indexing
    shift-right: [w84] -> _
    shift-left: w23 -> [w138]
    shift-right: [w115] -> _
    shift-left: w21 -> [w125]
    shift-right: [w116] -> _
    shift-left: w19 -> [w118]
    shift-right: [w78] -> _
    shift-left: w23 -> [w106]
    shift-right: [w79] -> _
    shift-left: w23 -> [w105]
    shift-right: [w83] -> _
    shift-left: w23 -> [w94]
    shift-right: [w82] -> _
    shift-left: w23 -> [w93]
    shift-right: [w76] -> _
    shift-left: w23 -> [w92]
    shift-right: [w86] -> _
    shift-left: w23 -> [w91]
    shift-right: [w77] -> _
    shift-left: w23 -> [w90]
    shift-right: [w75] -> _
    shift-left: w23 -> [w89]
    shift-right: [w81] -> _
    shift-left: w23 -> [w88]
    shift-right: [w80] -> _
    shift-left: w23 -> [w87]
    shift-right: [w66] -> w2
    shift-left: "SMU4" -> [w168]
    i -> [w128]
    stop <- "Interrupt program" stop-if-true
    # "Is off"
    # "Is on"
    # "Ig off"
    # "Ig on"
    # "Is min"
    # "Is max"
    # "Ig min"
    # "Ig max"
    # "Id min"
    # "Id max"
    # "Id off"
    # "Id on"
    # "Is off"
    # "Is on"
    # "Ig off"
    # "Ig on"
    # "Is min"
    # "Is max"
    # "Ig min"
    # "Ig max"
    # "Id min"
    # "Id max"
    # "Id off"
    # "Id on"
    # "Filepath and name"
    # "Limit of command arguments (array columns). Raise if needed."
    # "Serial port data (string)"
    # "Serial port data (table)"
    # "Serial port data"
    # "For loop counter"
    # "<-----Equivalent to the 4155C \"Write\" subvi.----->"
    # "Headers"
    # "Save transfer curves in file."
    # "Filepath and name"
    # "Save time-dependent data."
    # "Use the time offset if your measurements do not start at t=0."
    # "Time for Imax, Imin, Ion, Ioff"
    # "Rest of elements of command"
    # "First element of command\n(case select)"
    n20 = Add(x=w128, y=1) -> (x+y=→"Line running":i32)
    n21 = Add(x=w133, y=1) -> (x+y=→"Total lines":i32)
    n22 = Index Array(array=w161, index=0 ("line index")) -> (element=w156:string)
    "Command running:" <- w156
    n23 = control-ref of="Interrupt scan"() -> (w180:refnum<vi>)
    n24 = Spreadsheet String To Array(delimiter (Tab)=" ", format string="%s", spreadsheet string=w156, array type (2D Dbl)=string[] []) -> (array=w154:string[])
    n25 = Delete From Array(array=w154, index=0) -> (deleted portion=w107:string, array with subset deleted=w153:string[])  [unwired: 1 in]
    n26 = call "Elapsed Time"("Reset"="Reset", "Auto Reset"="Auto Reset") -> ("Elapsed Time (s)"=w163:dbl)  [unwired: 10 in, 7 out]
    n27 = case shown="2" "Time Units" {
      tunnel: ["-sec" "-min" "-h"] -> w164
      tunnel: [w194 w198 w201] -> w134
      tunnel: w163 -> [w194 w197 w202]
      frame 0, Default {
      }
      frame 1 {
        n28 = Divide(x=w197, y=60.0) -> (x/y=w198:dbl)
      }
      frame 2 {
        n29 = Divide(x=w202, y=3600.0) -> (x/y=w201:dbl)
      }
    }
    n30 = Add(x=w134, y="Time Offset") -> (x+y=w64:dbl)
    n31 = To Long Integer(number=w64) -> (32bit integer=w65:i32)
    "Elapsed Time" <- w65
    n32 = case shown="\"sample\"" w107 {
      tunnel: w153 -> [w234 w267 w299 w311 w428 w535 w670 w785 w941 w969 w1038 w1079 w1118 w1153 w1181 _ _ w1345 w1461 _ w1554 w1612 w1668 w1752 w1828 w1862]
      tunnel: w190 -> [w229 w263 w297 w324 w435 w594 w678 w792 w949 w986 w1027 w1071 w1111 w1147 w1174 w1207 w1263 w1326 w1443 w1488 w1541 w1599 w1656 w1746 w1824 w1864]
      tunnel: w189 -> [w228 w262 w288 w323 w406 w579 w647 w763 w917 w987 w1028 w1072 w1112 w1148 w1175 w1212 w1265 w1351 w1467 w1492 w1560 w1618 w1674 w1758 w1782 w1868]
      tunnel: w188 -> [w227 w261 w287 w322 w405 w578 w646 w762 w914 w988 w1029 w1073 w1113 w1149 w1176 w1211 w1236 w1350 w1466 w1491 w1559 w1617 w1673 w1757 w1781 w1867]
      tunnel: w187 -> [w226 w260 w296 w320 w431 w555 w674 w788 w945 w996 w1037 w1070 w1110 w1146 w1173 w1210 w1260 w1318 w1435 w1497 w1534 w1592 w1649 w1745 w1823 w1869]
      tunnel: w186 -> [w225 w259 w295 w319 w433 w592 w676 w790 w947 w995 w1036 w1078 w1117 w1152 w1180 w1209 w1245 w1349 w1465 w1500 w1558 w1616 w1672 w1756 w1832 w1870]
      tunnel: w185 -> [w224 w258 w294 w317 w432 w591 w675 w789 w946 w994 w1035 w1077 w1116 w1151 w1179 w1208 w1246 w1327 w1444 w1499 w1542 w1600 w1657 w1747 w1825 w1872]
      tunnel: [w228 w262 w286 w323 w430 w589 w672 w787 w943 w987 w1028 w1072 w1112 w1148 w1175 w1212 w1265 w1319 w1417 w1490 w1535 w1593 w1650 w1698 w1784 w1868] -> w184
      tunnel: [w227 w261 w285 w322 w429 w588 w671 w786 w942 w988 w1029 w1073 w1113 w1149 w1176 w1211 w1235 w1328 w1418 w1489 w1543 w1601 w1658 w1697 w1783 w1866] -> w119
      tunnel: [w226 w260 w296 w320 w431 w551 w674 w788 w945 w989 w1030 w1070 w1110 w1146 w1173 w1210 w1260 w1318 w1435 w1497 w1534 w1592 w1649 w1745 w1823 w1869] -> w183
      tunnel: [w225 w259 w295 w319 w433 w592 w676 w790 w947 w995 w1036 w1078 w1117 w1152 w1180 w1209 w1245 w1349 w1465 w1500 w1558 w1616 w1672 w1756 w1832 w1870] -> w182
      tunnel: [w224 w258 w294 w317 w432 w591 w675 w789 w946 w994 w1035 w1077 w1116 w1151 w1179 w1208 w1246 w1327 w1444 w1499 w1542 w1600 w1657 w1747 w1825 w1872] -> w181
      tunnel: [w229 w263 w297 w324 w435 w594 w678 w792 w949 w986 w1027 w1071 w1111 w1147 w1174 w1207 w1263 w1326 w1443 w1488 w1541 w1599 w1656 w1746 w1824 w1864] -> w73
      tunnel: w180 -> [_ _ _ _ w437 w598 w683 w794 w953 _ _ _ _ _ _ _ _ w1323 w1440 _ w1540 w1598 w1655 w1718 w1800 _]
      tunnel: "Gate" -> [_ _ _ _ w415 w582 w657 w772 w928 _ _ _ _ _ _ _ _ _ _ _ _ _ _ _ _ _]
      tunnel: "Drain 2" -> [_ _ _ _ w414 w581 w656 w771 w927 _ _ _ _ _ _ _ _ _ _ _ _ _ _ _ _ _]
      tunnel: "Panel Controls" -> [_ _ _ _ _ _ w655 w698 w926 _ _ _ _ _ _ _ _ _ _ _ _ _ _ _ _ _]
      tunnel: w176 -> [w223 w257 w293 w316 w399 w572 w640 w756 w912 w993 w1034 _ w1109 w1145 w1172 w1206 w1247 w1314 w1431 w1493 w1530 w1588 w1645 w1741 w1819 w1873]
      tunnel: w175 -> [w222 w256 w292 w315 w398 w571 w639 w755 w911 w992 w1033 w1076 _ w1136 w1178 w1205 w1248 w1315 w1432 w1494 w1531 w1589 w1646 w1742 w1820 w1874]
      tunnel: w174 -> [w221 w255 w291 w314 w397 w570 w638 w754 w910 w991 w1032 w1075 w1115 w1150 _ w1204 w1249 w1316 w1433 w1495 w1532 w1590 w1647 w1743 w1821 w1875]
      tunnel: w173 -> [w220 w254 w290 w313 w396 w569 w637 w753 w913 w990 w1031 w1074 w1114 _ w1177 w1203 w1250 w1317 w1434 w1496 w1533 w1591 w1648 w1744 w1822 w1876]
      tunnel: [w223 w257 w293 w316 w399 w572 w640 w756 w912 w993 w1034 w1069 w1109 w1145 w1172 w1206 w1247 w1314 w1431 w1493 w1530 w1588 w1645 w1741 w1819 w1873] -> w172
      tunnel: [w222 w256 w292 w315 w398 w571 w639 w755 w911 w992 w1033 w1076 w1101 w1136 w1178 w1205 w1248 w1315 w1432 w1494 w1531 w1589 w1646 w1742 w1820 w1874] -> w171
      tunnel: [w221 w255 w291 w314 w397 w570 w638 w754 w910 w991 w1032 w1075 w1115 w1150 w1171 w1204 w1249 w1316 w1433 w1495 w1532 w1590 w1647 w1743 w1821 w1875] -> w170
      tunnel: [w220 w254 w290 w313 w396 w569 w637 w753 w913 w990 w1031 w1074 w1114 w1137 w1177 w1203 w1250 w1317 w1434 w1496 w1533 w1591 w1648 w1744 w1822 w1876] -> w169
      tunnel: w168 -> [w204 w235 w268 _ w337 w524 w609 w694 w881 w966 w1010 w1053 w1085 w1120 w1155 w1187 w1213 w1301 w1397 w1472 w1501 w1563 w1621 w1677 w1759 w1833]
      tunnel: w167 -> [_ _ _ _ w390 w566 _ _ _ _ _ _ _ _ _ _ _ _ _ _ _ _ _ _ _ _]
      tunnel: [w219 w250 w283 w328 w352 w543 w627 w710 w899 w985 w1025 w1068 w1100 w1135 w1170 w1202 w1231 w1291 w1401 w1487 w1519 w1581 w1639 w1695 w1777 w1865] -> w85
      tunnel: w166 -> [w219 w250 w283 w328 w387 w543 w627 w745 w899 w985 w1025 w1068 w1100 w1135 w1170 w1202 w1231 w1297 w1401 w1487 w1519 w1581 w1639 w1695 w1777 w1865]
      tunnel: w64 -> [_ _ _ _ w386 w540 w625 w744 w896 _ _ _ _ _ _ _ w1229 w1306 w1413 _ w1516 w1578 w1636 w1692 w1773 _]
      tunnel: w164 -> [_ _ _ _ w383 w539 w623 w741 w895 _ _ _ _ _ _ _ w1227 w1304 w1412 _ w1515 w1577 w1635 w1691 w1774 _]
      tunnel: w65 -> [_ _ _ _ w379 _ _ w737 _ _ _ _ _ _ _ _ _ _ _ _ _ _ _ _ _ _]
      tunnel: [w218 w249 w282 w318 w356 w542 w626 w714 w898 w984 w1024 w1067 w1099 w1134 w1169 w1201 w1230 w1273 w1415 w1486 w1518 w1580 w1638 w1694 w1776 w1871] -> w120
      tunnel: w162 -> [w218 w249 w282 w318 w382 w542 w626 w740 w898 w984 w1024 w1067 w1099 w1134 w1169 w1201 w1230 w1275 w1415 w1486 w1518 w1580 w1638 w1694 w1776 w1871]
      tunnel: [w217 w248 w281 w327 w351 w538 w622 w709 w894 w983 w1023 w1066 w1098 w1133 w1168 w1200 w1226 w1290 w1400 w1485 w1514 w1576 w1634 w1690 w1772 w1860] -> w84
      tunnel: w138 -> [w217 w248 w281 w327 w378 w538 w622 w736 w894 w983 w1023 w1066 w1098 w1133 w1168 w1200 w1226 w1296 w1400 w1485 w1514 w1576 w1634 w1690 w1772 w1860]
      tunnel: [w216 w247 w280 w312 w371 w537 w621 w729 w893 w982 w1022 w1065 w1097 w1132 w1167 w1199 w1225 w1303 w1411 w1484 w1513 w1575 w1633 w1689 w1771 w1859] -> w115
      tunnel: w125 -> [w216 w247 w280 w312 w371 w537 w621 w729 w893 w982 w1022 w1065 w1097 w1132 w1167 w1199 w1225 w1303 w1411 w1484 w1513 w1575 w1633 w1689 w1771 w1858]
      tunnel: [w215 w246 w279 w321 w370 w536 w620 w728 w892 w981 w1021 w1064 w1096 w1131 w1166 w1198 w1224 w1302 w1410 w1483 w1512 w1574 w1632 w1688 w1770 w1844] -> w116
      tunnel: w118 -> [w215 w246 w279 w321 w370 w536 w620 w728 w892 w981 w1021 w1064 w1096 w1131 w1166 w1198 w1224 w1302 w1410 w1483 w1512 w1574 w1632 w1688 w1770 w1844]
      tunnel: [w213 w244 w277 w333 w345 w533 w618 w703 w890 w979 w1020 w1063 w1094 w1129 w1164 w1196 w1222 w1284 w1409 w1482 w1511 w1573 w1630 w1687 w1769 w1843] -> w78
      tunnel: w106 -> [w213 w244 w277 w333 w369 w533 w618 w727 w890 w979 w1020 w1063 w1094 w1129 w1164 w1196 w1222 w1284 w1409 w1482 w1511 w1573 w1630 w1687 w1769 w1843]
      tunnel: [w214 w245 w278 w334 w346 w534 w619 w704 w891 w980 w1019 w1062 w1095 w1130 w1165 w1197 w1223 w1285 w1408 w1481 w1510 w1572 w1631 w1686 w1768 w1842] -> w79
      tunnel: w105 -> [w214 w245 w278 w334 w368 w534 w619 w726 w891 w980 w1019 w1062 w1095 w1130 w1165 w1197 w1223 w1285 w1408 w1481 w1510 w1572 w1631 w1686 w1768 w1842]
      tunnel: [w206 w237 w270 w326 w350 w530 w616 w708 w888 w972 w1017 w1060 w1092 w1127 w1162 w1194 w1215 w1289 w1399 w1480 w1503 w1565 w1623 w1679 w1763 w1835] -> w83
      tunnel: w94 -> [w206 w237 w270 w326 w364 w530 w616 w722 w888 w972 w1017 w1060 w1092 w1127 w1162 w1194 w1215 w1295 w1399 w1480 w1503 w1565 w1623 w1679 w1763 w1835]
      tunnel: [w205 w236 w269 w325 w349 w531 w617 w707 w889 w971 w1018 w1061 w1093 w1128 w1163 w1195 w1214 w1288 w1398 w1479 w1502 w1564 w1622 w1678 w1762 w1834] -> w82
      tunnel: w93 -> [w205 w236 w269 w325 w363 w531 w617 w721 w889 w971 w1018 w1061 w1093 w1128 w1163 w1195 w1214 w1294 w1398 w1479 w1502 w1564 w1622 w1678 w1762 w1834]
      tunnel: [w208 w239 w272 w330 w355 w529 w614 w713 w886 w977 w1015 w1058 w1090 w1125 w1160 w1192 w1217 w1293 w1403 w1474 w1505 w1567 w1625 w1681 w1761 w1839] -> w76
      tunnel: w92 -> [w208 w239 w272 w330 w362 w529 w614 w720 w886 w977 w1015 w1058 w1090 w1125 w1160 w1192 w1217 w1299 w1403 w1474 w1505 w1567 w1625 w1681 w1761 w1839]
      tunnel: [w207 w238 w271 w329 w353 w532 w615 w711 w887 w978 w1016 w1059 w1091 w1126 w1161 w1193 w1216 w1292 w1402 w1473 w1504 w1566 w1624 w1680 w1760 w1838] -> w86
      tunnel: w91 -> [w207 w238 w271 w329 w361 w532 w615 w719 w887 w978 w1016 w1059 w1091 w1126 w1161 w1193 w1216 w1298 w1402 w1473 w1504 w1566 w1624 w1680 w1760 w1838]
      tunnel: [w210 w241 w274 w332 w344 w528 w612 w702 w884 w975 w1013 w1056 w1088 w1123 w1158 w1190 w1219 w1283 w1405 w1476 w1507 w1569 w1627 w1683 w1765 w1841] -> w77
      tunnel: w90 -> [w210 w241 w274 w332 w360 w528 w612 w718 w884 w975 w1013 w1056 w1088 w1123 w1158 w1190 w1219 w1283 w1405 w1476 w1507 w1569 w1627 w1683 w1765 w1841]
      tunnel: [w209 w240 w273 w331 w343 w527 w613 w701 w885 w976 w1014 w1057 w1089 w1124 w1159 w1191 w1218 w1282 w1404 w1475 w1506 w1568 w1626 w1682 w1764 w1840] -> w75
      tunnel: w89 -> [w209 w240 w273 w331 w359 w527 w613 w717 w885 w976 w1014 w1057 w1089 w1124 w1159 w1191 w1218 w1282 w1404 w1475 w1506 w1568 w1626 w1682 w1764 w1840]
      tunnel: [w212 w243 w276 w336 w348 w526 w610 w706 w882 w973 w1011 w1054 w1086 w1121 w1156 w1188 w1221 w1287 w1407 w1478 w1509 w1571 w1629 w1685 w1767 w1837] -> w81
      tunnel: w88 -> [w212 w243 w276 w336 w358 w526 w610 w716 w882 w973 w1011 w1054 w1086 w1121 w1156 w1188 w1221 w1287 w1407 w1478 w1509 w1571 w1629 w1685 w1767 w1837]
      tunnel: [w211 w242 w275 w335 w347 w525 w611 w705 w883 w974 w1012 w1055 w1087 w1122 w1157 w1189 w1220 w1286 w1406 w1477 w1508 w1570 w1628 w1684 w1766 w1836] -> w80
      tunnel: w87 -> [w211 w242 w275 w335 w357 w525 w611 w715 w883 w974 w1012 w1055 w1087 w1122 w1157 w1189 w1220 w1286 w1406 w1477 w1508 w1570 w1628 w1684 w1766 w1836]
      tunnel: [w204 w235 w268 w302 w337 w524 w609 w694 w881 w966 w1010 w1053 w1085 w1120 w1155 w1187 w1213 w1301 w1397 w1472 w1501 w1563 w1621 w1677 w1759 w1833] -> w66
      tunnel: w64 -> [_ _ _ _ _ _ _ _ _ _ _ _ _ _ _ _ _ w1266 _ _ _ _ _ _ _ _]
      frame "wait" {
        n33 = Index Array(array=w234, index=0 ("Index")) -> (element=w232:string)
        n34 = Decimal String To Number(string=w232, default (0L)=u32 0) -> (number=w231:u32)  [unwired: 1 in, 1 out]
        n35 = Wait (ms)(milliseconds to wait=w231) -> ()  [unwired: 1 out]
      }
      frame "wait-min" {
        n36 = Index Array(array=w267, index=0 ("Index")) -> (element=w265:string)
        n37 = Decimal String To Number(string=w265, default (0L)=u32 0) -> (number=w253:u32)  [unwired: 1 in, 1 out]
        n38 = Multiply(x=w253, y=u32 60000) -> (x*y=w252:u32)
        n39 = Wait (ms)(milliseconds to wait=w252) -> ()  [unwired: 1 out]
      }
      frame "standby" {
        n40 = Index Array(array=w299, index=0 ("Index")) -> (element=w289:string)
        n41 = case shown="\"off\", Default" w289 {
          tunnel: [":PAGE:SCON:STAN 0" ":PAGE:SCON:STAN 1"] -> w284
          frame "off", Default {
          }
          frame "on" {
          }
        }
        n42 = VISA Write(VISA resource name=w288, write buffer=w284, error in (no error)=w287) -> (VISA resource name out=w286:refnum<visa-resource-name>, error out=w285:errorcluster)  [unwired: 1 out]
      }
      frame "SMU4" {
        n43 = Delete From Array(array=w311, index=0) -> (deleted portion=w305:string, array with subset deleted=w308:string[])  [unwired: 1 in]
        n44 = Equal?(x=w305, y="ON") -> (x = y?=w303:bool)
        n45 = Delete From Array(array=w308, index=0) -> (deleted portion=w307:string)  [unwired: 1 in, 1 out]
        n46 = Fract/Exp String To Number(string=w307) -> (number=w304:dbl)  [unwired: 3 in, 1 out]
        n47 = Bundle(w303, w304) -> (w302:cluster{bool, dbl})  [unwired: 1 in]
      }
      frame "transfer" {
        n48 = Delete From Array(array=w428, index=0 ("Index")) -> (deleted portion=w426:string, array with subset deleted=w425:string[])  [unwired: 1 in]
        n49 = Bundle By Name(cluster=w390, "Emergency Stop"=w437) -> (w391:T2)
        n50 = Number To Decimal String(number=w386) -> (decimal integer string=w385:string)  [unwired: 1 in]
        n51 = case shown="\"d\", Default" w426 {
          tunnel: [w522 w523] -> w424
          frame "s" {
            w522 = u16 0 items=["Single", "Double"] ("sweep mode")
          }
          frame "d", Default {
            w523 = u16 1 items=["Single", "Double"] ("sweep mode")
          }
        }
        n52 = Fract/Exp String To Number(string=w425) -> (number=w410:dbl[])  [unwired: 3 in, 1 out]
        n53 = Concatenate Strings(w435, "-transfer-" ("Prefix"), w385, w383, ".txt" ("Suffix (transfer)")) -> (w436:string)
        n54 = VISA Write(VISA resource name=w406, write buffer=":PAGE:CHAN:MODE SWE;" ("write buffer (\"\")"), error in (no error)=w405) -> (VISA resource name out=w403:refnum<visa-resource-name>, error out=w404:errorcluster)  [unwired: 1 out]
        n55 = local read "Plot transfer curve extrema vs time"() -> (w338:bool)
        n56 = String To Path(string=w436) -> (path=w434:path)
        n57 = Index Array(array=w410, index #1=0 ("Index")) -> (element #1=w423:dbl, element #2=w422:dbl, element #3=w421:dbl)  [unwired: 2 in]
        n58 = Delete From Array(array=w410, length=3 ("Length"), index=0 ("Index")) -> (array with subset deleted=w408:dbl[])  [unwired: 1 out]
        n59 = case shown="True" w338 {
          tunnel: w382 -> [w439 w442]
          tunnel: w379 -> [_ w441]
          tunnel: [w439 w440] -> w356
          frame False {
          }
          frame True {
            n60 = Build Array (concatenate)(w442, w441) -> (w440:i32[])
          }
        }
        n61 = Bundle By Name(cluster=w415, "Gate Start"=w423, "Gate Stop"=w422, "Gate Step (linear only)"=w421, "Gate Compliance"=w432, "Range mode"=w399, "Range"=w398) -> (w400:T6)
        n62 = Index Array(array=w408, index #1=0 ("Index")) -> (element #1=w418:dbl, element #2=w417:dbl, element #3=w416:dbl)  [unwired: 2 in]
        n63 = call <vilib>:"compatOverwrite.vi"("overwrite (F)"=TRUE) -> ("overwrite?"=w389:T8)
        n64 = Bundle By Name(cluster=w414, "Drain Start"=w418, "Drain Stop"=w417, "Drain Step"=w416, "Drain Compliance"=w433, "Range mode"=w397, "Range"=w396) -> (w401:T7)
        n65 = call "4155C Transfer.vi"("VISA resource name in"=w403, "Gate"=w400, "Drain"=w401, "Timings"=w431, "error in (no error)"=w404, "SMU4"=w337, "sweep mode"=w424, "Panel Controls"=w391) -> ("VG"=w388:dbl[], "Outparams"=w395:T9, "VISA Resource Name out"=w430:refnum<visa-resource-name>, "IS"=w366:dbl[], "ID"=w367:dbl[], "IG"=w365:dbl[], "error out"=w380:errorcluster, "SMU4"=w392:dbl[])  [unwired: 12 in]
        n66 = Unbundle By Name(w395) -> ("V2 Step"=w394:dbl, "V2 Start"=w393:dbl, "Number of points"=w354:i32)
        n67 = call "4155C Split array.vi"("Number of VAR2 steps"=w354, "Y2 data in"=w367, "X data in"=w388, "Y1 data in"=w366, "Y3 data in"=w365, "error in (no error)"=w380) -> ("Array of clusters"=w381:cluster{"Y data in":dbl[], "X data in":dbl[]}[], "error out"=w342:errorcluster)  [unwired: 1 in]
        n68 = case shown="True" "Plot transfer curve extrema vs time" {
          tunnel: w387 -> [w445 w521]
          tunnel: w378 -> [w446 w516]
          tunnel: w369 -> [w452 w512]
          tunnel: w368 -> [w453 w511]
          tunnel: w367 -> [_ w508]
          tunnel: w366 -> [_ w506]
          tunnel: w365 -> [_ w505]
          tunnel: w364 -> [w447 w501]
          tunnel: w363 -> [w449 w500]
          tunnel: w362 -> [w443 w497]
          tunnel: w361 -> [w444 w496]
          tunnel: w360 -> [w451 w493]
          tunnel: w359 -> [w450 w492]
          tunnel: w358 -> [w455 w489]
          tunnel: w357 -> [w454 w488]
          tunnel: w356 -> [_ w481]
          tunnel: [w443 w476] -> w355
          tunnel: w354 -> [_ w475]
          tunnel: [w444 w474] -> w353
          tunnel: [w445 w473] -> w352
          tunnel: [w446 w472] -> w351
          tunnel: [w447 w471] -> w350
          tunnel: [w449 w470] -> w349
          tunnel: [w455 w469] -> w348
          tunnel: [w454 w468] -> w347
          tunnel: [w453 w467] -> w346
          tunnel: [w452 w466] -> w345
          tunnel: [w451 w465] -> w344
          tunnel: [w450 w464] -> w343
          tunnel: w342 -> [w448 w463]
          tunnel: [w448 w459] -> w341
          frame False {
          }
          frame True {
            # "Adjusts graph colors."
            # "Adjusts graph colors."
            # "Ion will be the middle element of the array. The calculation of the index is done only once, since Is, Id, and Ig have the same dimensions."
            # "abs(Ig)"
            # "abs(Is)"
            # "Y1: Is\nY2: Id\nY3: Ig"
            # "abs(Id)"
            # "Adjusts graph colors."
            # "Adjusts graph colors."
            # "Adjusts graph colors."
            n69 = Absolute Value(x=w506) -> (abs(x)=w491:dbl[])
            n70 = Absolute Value(x=w508) -> (abs(x)=w507:dbl[])
            n71 = Absolute Value(x=w505) -> (abs(x)=w494:dbl[])
            n72 = Array Size(array=w507) -> (size(s)=w515:i32)
            n73 = Divide(x=w515, y=2) -> (x/y=w458:dbl)
            n74 = Subtract(x=w458, y=1) -> (x-y=w457:dbl)
            n75 = Array Max & Min(array=w491) -> (max value=w498:dbl, min value=w499:dbl)  [unwired: 2 out]
            n76 = Array Max & Min(array=w507) -> (max value=w520:dbl, min value=w504:dbl)  [unwired: 2 out]
            n77 = Array Max & Min(array=w494) -> (max value=w503:dbl, min value=w502:dbl)  [unwired: 2 out]
            n78 = Index Array(array=w491, index=w457) -> (element=w482:dbl)
            n79 = Index Array(array=w491, index=0) -> (element=w483:dbl)
            n80 = Index Array(array=w507, index=w457) -> (element=w484:dbl)
            n81 = Index Array(array=w507, index=0) -> (element=w485:dbl)
            n82 = Index Array(array=w494, index=w457) -> (element=w487:dbl)
            n83 = Index Array(array=w494, index=0) -> (element=w486:dbl)
            n84 = local write "Ig max"(w503) -> ()
            n85 = local write "Ig min"(w502) -> ()
            n86 = local write "Is max"(w498) -> ()
            n87 = local write "Is min"(w499) -> ()
            n88 = local write "Id max"(w520) -> ()
            n89 = local write "Id min"(w504) -> ()
            n90 = Build Array (concatenate)(w497, w498) -> (w476:dbl[])
            n91 = Build Array (concatenate)(w496, w499) -> (w474:dbl[])
            n92 = local write "Is off"(w483) -> ()
            n93 = local write "Is on"(w482) -> ()
            n94 = Build Array (concatenate)(w521, w520) -> (w473:dbl[])
            n95 = Build Array (concatenate)(w516, w504) -> (w472:dbl[])
            n96 = Build Array (concatenate)(w501, w503) -> (w471:dbl[])
            n97 = Build Array (concatenate)(w500, w502) -> (w470:dbl[])
            n98 = Build Array (concatenate)(w489, w482) -> (w469:dbl[])
            n99 = Build Array (concatenate)(w488, w483) -> (w468:dbl[])
            n100 = Build Array (concatenate)(w511, w484) -> (w467:dbl[])
            n101 = Build Array (concatenate)(w512, w485) -> (w466:dbl[])
            n102 = Build Array (concatenate)(w493, w487) -> (w465:dbl[])
            n103 = Build Array (concatenate)(w492, w486) -> (w464:dbl[])
            n104 = local write "Ig off"(w486) -> ()
            n105 = local write "Ig on"(w487) -> ()
            n106 = local write "Id off"(w485) -> ()
            n107 = local write "Id on"(w484) -> ()
            n108 = control-ref of="Imax vs time"() -> (w510:refnum<vi>)
            n109 = control-ref of="Imin vs time"() -> (w509:refnum<vi>)
            n110 = control-ref of="Ion vs time"() -> (w478:refnum<vi>)
            n111 = control-ref of="Ioff vs time"() -> (w477:refnum<vi>)
            n112 = control-ref of="I vs Vg"() -> (w519:refnum<vi>)
            n113 = call "4155C Split array.vi"("Number of VAR2 steps"=w475, "Y2 data in"=w467, "X data in"=w481, "Y1 data in"=w469, "Y3 data in"=w465, "error in (no error)"=w463) -> ("Array of clusters"=w479:cluster{"Y data in":dbl[], "X data in":dbl[]}[], "error out"=w462:errorcluster)  [unwired: 1 in]
            n114 = call "4155C Split array.vi"("Number of VAR2 steps"=w475, "Y2 data in"=w466, "X data in"=w481, "Y1 data in"=w468, "Y3 data in"=w464, "error in (no error)"=w462) -> ("Array of clusters"=w480:cluster{"Y data in":dbl[], "X data in":dbl[]}[], "error out"=w461:errorcluster)  [unwired: 1 in]
            n115 = call "4155C Split array.vi"("Number of VAR2 steps"=w475, "Y2 data in"=w473, "X data in"=w481, "Y1 data in"=w476, "Y3 data in"=w471, "error in (no error)"=w461) -> ("Array of clusters"=w518:cluster{"Y data in":dbl[], "X data in":dbl[]}[], "error out"=w460:errorcluster)  [unwired: 1 in]
            n116 = call "4155C Split array.vi"("Number of VAR2 steps"=w475, "Y2 data in"=w472, "X data in"=w481, "Y1 data in"=w474, "Y3 data in"=w470, "error in (no error)"=w460) -> ("Array of clusters"=w517:cluster{"Y data in":dbl[], "X data in":dbl[]}[], "error out"=w459:errorcluster)  [unwired: 1 in]
            n117 = call "4155C Config Chart Colours.vi"("Numeric"=w475, "XY Graph 2"=w510) -> ()  [unwired: 6 in]
            n118 = call "4155C Config Chart Colours.vi"("Numeric"=w475, "XY Graph 2"=w509) -> ()  [unwired: 6 in]
            n119 = call "4155C Config Chart Colours.vi"("Numeric"=w475, "XY Graph 2"=w478) -> ()  [unwired: 6 in]
            n120 = call "4155C Config Chart Colours.vi"("Numeric"=w475, "XY Graph 2"=w477) -> ()  [unwired: 6 in]
            n121 = call "4155C Config Chart Colours.vi"("Numeric"=w475, "XY Graph 2"=w519) -> ()  [unwired: 6 in]
            n122 = local write "Imax vs time"(w518) -> ()
            n123 = local write "Imin vs time"(w517) -> ()
            n124 = local write "Ion vs time"(w479) -> ()
            n125 = local write "Ioff vs time"(w480) -> ()
          }
        }
        n126 = local write "I vs Vg"(w381) -> ()
        n127 = Open/Create/Replace File(file path (use dialog)=w434, error in=w341, operation (0:open)=w389) -> (refnum out=w376:refnum<file>, error out=w374:errorcluster)  [unwired: 3 in, 1 out]
        n128 = call "4155C Make Big 2d array.vi"("1D Var1"=w388, "1d IS"=w366, "1d ID"=w367, "1d IG"=w365, "1d SMU4"=w392, "SMU4"=w337, "VAR2 START"=w393, "Number of VAR2 steps"=w354, "VAR2 STEP"=w394, "VAR1 Name"="Vg", "Decimal places in header"=i8 1, "VAR2 Name"="Vd") -> ("Header array"=w377:string[], "Data array"=w375:dbl[][])  [unwired: 14 in]
        n129 = call "4155C Write array to file.vi"("Byte Stream File Refnum"=w376, "Header"=w377, "Data Array"=w375, "error in (no error)"=w374) -> ("dup refnum"=w373:refnum<file>, "error out"=w372:errorcluster)  [unwired: 1 in]
        n130 = Close File(refnum=w373, error in=w372) -> (error out=w429:errorcluster)  [unwired: 1 out]
      }
      frame "pulsedstressV" {
        w549 = 0
        n131 = Number To Decimal String(number=w540) -> (decimal integer string=w595:string)  [unwired: 1 in]
        n132 = Delete From Array(array=w535, index=0 ("Index")) -> (deleted portion=w586:string, array with subset deleted=w585:string[])  [unwired: 1 in]
        n133 = Bundle By Name(cluster=w566, "Emergency Stop"=w598) -> (w567:T2)
        n134 = VISA Write(VISA resource name=w579, write buffer=":PAGE:CHAN:MODE SWE;" ("write buffer (\"\")"), error in (no error)=w578) -> (VISA resource name out=w576:refnum<visa-resource-name>, error out=w577:errorcluster)  [unwired: 1 out]
        n135 = Concatenate Strings(w594, "-pulsedstressV-" ("Substring"), w595, w539, ".txt" ("Substring")) -> (w597:string)
        n136 = case shown="\"d\", Default" w586 {
          tunnel: [w607 w608] -> w584
          frame "s" {
            w607 = u16 0 items=["Single", "Double"] ("sweep mode")
          }
          frame "d", Default {
            w608 = u16 1 items=["Single", "Double"] ("sweep mode")
          }
        }
        n137 = Fract/Exp String To Number(string=w585) -> (number=w580:dbl[])  [unwired: 3 in, 1 out]
        n138 = String To Path(string=w597) -> (path=w593:path)
        n139 = Index Array(array=w580, index #1=0 ("Index")) -> (element #1=w558:dbl, element #2=w557:dbl, element #3=w554:dbl, element #4=w553:dbl, element #5=w552:dbl, element #6=w556:dbl)  [unwired: 5 in]
        n140 = Bundle By Name(cluster=w555, "Pulse period"=w553, "Base voltage"=w554, "Pulse width"=w552) -> (w551:T4)
        n141 = Unbundle By Name(w551) -> ("Pulse period"=w559:dbl)
        n142 = Bundle By Name(cluster=w582, "Gate Start"=w557, "Gate Stop"=w558, "Gate Step (linear only)"=0, "Gate Compliance"=w591, "Range mode"=w572, "Range"=w571) -> (w573:T6)
        n143 = call <vilib>:"compatOverwrite.vi"("overwrite (F)"=TRUE) -> ("overwrite?"=w544:T8)
        n144 = Bundle By Name(cluster=w581, "Drain Start"=w556, "Drain Stop"=w549, "Drain Step"=w549, "Drain Compliance"=w592, "Range mode"=w570, "Range"=w569) -> (w574:T7)
        n145 = call "4155C PulsedStressV.vi"("VISA resource name in"=w576, "sweep mode"=w584, "Panel Controls"=w567, "Gate"=w573, "Drain"=w574, "Timings"=w551, "error in (no error)"=w577, "SMU4"=w524) -> ("VISA Resource Name out"=w589:refnum<visa-resource-name>, "ID"=w547:dbl[], "IG"=w545:dbl[], "Outparams"=w568:T9, "error out"=w590:errorcluster)  [unwired: 3 in]
        n146 = Unbundle By Name(w568) -> ("Number of points"=w546:i32)  [unwired: 2 out]
        n147 = for {
          N: w546 -> [_]
          tunnel: [w604] -> w548 mode=indexing
          tunnel: w559 -> [w606]
          i -> [w605]
          n148 = Multiply(x=w606, y=w605) -> (x*y=w604:dbl)
        }
        n149 = Insert Into Array(array=dbl[][] [] ("Input Array"), new element=w548) -> (w560:dbl[][])  [unwired: 2 in]
        n150 = Insert Into Array(array=w560, new element=w547) -> (w565:dbl[][])  [unwired: 2 in]
        n151 = Insert Into Array(array=w565, new element=w545) -> (w564:dbl[][])  [unwired: 2 in]
        n152 = Transpose 2D Array(2D array=w564) -> (transposed array=w563:dbl[][])
        n153 = Open/Create/Replace File(file path (use dialog)=w593, error in=w590, operation (0:open)=w544) -> (refnum out=w601:refnum<file>, error out=w602:errorcluster)  [unwired: 3 in, 1 out]
        n154 = call "4155C Write array to file.vi"("Byte Stream File Refnum"=w601, "Header"=string[] ["Time /s", "Id /A", "Ig /A"], "Data Array"=w563, "error in (no error)"=w602) -> ("dup refnum"=w599:refnum<file>, "error out"=w600:errorcluster)  [unwired: 1 in]
        n155 = Close File(refnum=w599, error in=w600) -> (error out=w588:errorcluster)  [unwired: 1 out]
      }
      frame "transfer-fpp" {
        n156 = Number To Decimal String(number=w625) -> (decimal integer string=w679:string)  [unwired: 1 in]
        n157 = Bundle By Name(cluster=w655, "Emergency Stop"=w683) -> (w691:T1)
        n158 = Delete From Array(array=w670, index=0 ("Index")) -> (deleted portion=w668:string, array with subset deleted=w667:string[])  [unwired: 1 in]
        n159 = Concatenate Strings(w678, "-transferfpp-" ("Substring"), w679, w623, ".txt" ("Substring")) -> (w681:string)
        n160 = VISA Write(VISA resource name=w647, write buffer=":PAGE:CHAN:MODE SWE;" ("write buffer (\"\")"), error in (no error)=w646) -> (VISA resource name out=w644:refnum<visa-resource-name>, error out=w645:errorcluster)  [unwired: 1 out]
        n161 = case shown="\"d\", Default" w668 {
          tunnel: [w692 w693] -> w666
          frame "s" {
            w692 = u16 0 items=["Single", "Double"] ("sweep mode")
          }
          frame "d", Default {
            w693 = u16 1 items=["Single", "Double"] ("sweep mode")
          }
        }
        n162 = Fract/Exp String To Number(string=w667) -> (number=w651:dbl[])  [unwired: 3 in, 1 out]
        n163 = String To Path(string=w681) -> (path=w677:path)
        n164 = Index Array(array=w651, index #1=0 ("Index")) -> (element #1=w665:dbl, element #2=w664:dbl, element #3=w663:dbl)  [unwired: 2 in]
        n165 = Delete From Array(array=w651, length=3 ("Length"), index=0 ("Index")) -> (array with subset deleted=w649:dbl[])  [unwired: 1 out]
        n166 = Bundle By Name(cluster=w657, "Gate Start"=w665, "Gate Stop"=w664, "Gate Step (linear only)"=w663, "Gate Compliance"=w675, "Range mode"=w640, "Range"=w639) -> (w641:T6)
        n167 = Index Array(array=w649, index #1=0 ("Index")) -> (element #1=w660:dbl, element #2=w659:dbl, element #3=w658:dbl)  [unwired: 2 in]
        n168 = call <vilib>:"compatOverwrite.vi"("overwrite (F)"=TRUE) -> ("overwrite?"=w628:T8)
        n169 = Bundle By Name(cluster=w656, "Drain Start"=w660, "Drain Stop"=w659, "Drain Step"=w658, "Drain Compliance"=w676, "Range mode"=w638, "Range"=w637) -> (w642:T7)
        n170 = call "4155C Transfer-FPP.vi"("VISA resource name in"=w644, "Gate"=w641, "Drain"=w642, "Timings"=w674, "error in (no error)"=w645, "sweep mode"=w666, "Panel Controls"=w691) -> ("VG"=w682:dbl[], "Outparams"=w636:T9, "VISA Resource Name out"=w672:refnum<visa-resource-name>, "Vprobe2"=w632:dbl[], "ID"=w631:dbl[], "IG"=w630:dbl[], "Vprobe1"=w629:dbl[], "error out"=w673:errorcluster)  [unwired: 13 in]
        n171 = Unbundle By Name(w636) -> ("V2 Step"=w635:dbl, "V2 Start"=w634:dbl, "Number of points"=w633:i32)
        n172 = Open/Create/Replace File(file path (use dialog)=w677, error in=w673, operation (0:open)=w628) -> (refnum out=w688:refnum<file>, error out=w689:errorcluster)  [unwired: 3 in, 1 out]
        n173 = call "4155C Make Big 2d array FPP.vi"("1D Var1"=w682, "1d ID"=w631, "1d Vp2"=w632, "1d IG"=w630, "1d Vp1"=w629, "VAR2 START"=w634, "Number of VAR2 steps"=w633, "VAR2 STEP"=w635, "VAR1 Name"="Vg", "Decimal places in header"=i8 1, "VAR2 Name"="Vd") -> ("Header array"=w684:string[], "Data array"=w685:dbl[][])  [unwired: 15 in]
        n174 = call "4155C Write array to file.vi"("Byte Stream File Refnum"=w688, "Header"=w684, "Data Array"=w685, "error in (no error)"=w689) -> ("dup refnum"=w686:refnum<file>, "error out"=w687:errorcluster)  [unwired: 1 in]
        n175 = Close File(refnum=w686, error in=w687) -> (error out=w671:errorcluster)  [unwired: 1 out]
      }
      frame "output" {
        n176 = Delete From Array(array=w785, index=0 ("Index")) -> (deleted portion=w783:string, array with subset deleted=w782:string[])  [unwired: 1 in]
        n177 = Bundle By Name(cluster=w698, "Emergency Stop"=w794) -> (w748:T1)
        n178 = Number To Decimal String(number=w744) -> (decimal integer string=w743:string)  [unwired: 1 in]
        n179 = case shown="\"d\", Default" w783 {
          tunnel: [w879 w880] -> w781
          frame "s" {
            w879 = u16 0 items=["Single", "Double"] ("sweep mode")
          }
          frame "d", Default {
            w880 = u16 1 items=["Single", "Double"] ("sweep mode")
          }
        }
        n180 = Fract/Exp String To Number(string=w782) -> (number=w767:dbl[])  [unwired: 3 in, 1 out]
        n181 = Concatenate Strings(w792, "-output-" ("Substring"), w743, w741, ".txt" ("Suffix (transfer)")) -> (w793:string)
        n182 = VISA Write(VISA resource name=w763, write buffer=":PAGE:CHAN:MODE SWE;" ("write buffer (\"\")"), error in (no error)=w762) -> (VISA resource name out=w760:refnum<visa-resource-name>, error out=w761:errorcluster)  [unwired: 1 out]
        n183 = String To Path(string=w793) -> (path=w791:path)
        n184 = local read "Plot output curve extrema vs time"() -> (w695:bool)
        n185 = Index Array(array=w767, index #1=0 ("Index")) -> (element #1=w780:dbl, element #2=w779:dbl, element #3=w778:dbl)  [unwired: 2 in]
        n186 = Delete From Array(array=w767, length=3 ("Length"), index=0 ("Index")) -> (array with subset deleted=w765:dbl[])  [unwired: 1 out]
        n187 = case shown="True" w695 {
          tunnel: w740 -> [w796 w799]
          tunnel: w737 -> [_ w798]
          tunnel: [w796 w797] -> w714
          frame False {
          }
          frame True {
            n188 = Build Array (concatenate)(w799, w798) -> (w797:i32[])
          }
        }
        n189 = Bundle By Name(cluster=w772, "Gate Start"=w780, "Gate Stop"=w779, "Gate Step (linear only)"=w778, "Gate Compliance"=w789, "Range mode"=w756, "Range"=w755) -> (w757:T6)
        n190 = Index Array(array=w765, index #1=0 ("Index")) -> (element #1=w775:dbl, element #2=w774:dbl, element #3=w773:dbl)  [unwired: 2 in]
        n191 = call <vilib>:"compatOverwrite.vi"("overwrite (F)"=TRUE) -> ("overwrite?"=w747:T8)
        n192 = Bundle By Name(cluster=w771, "Drain Start"=w775, "Drain Stop"=w774, "Drain Step"=w773, "Drain Compliance"=w790, "Range mode"=w754, "Range"=w753) -> (w758:T7)
        n193 = call "4155C Output.vi"("VISA resource name in"=w760, "Gate"=w757, "Drain"=w758, "Timings"=w788, "error in (no error)"=w761, "SMU4"=w694, "sweep mode"=w781, "Panel controls"=w748) -> ("VD"=w746:dbl[], "Outparams"=w752:T9, "VISA Resource Name out"=w787:refnum<visa-resource-name>, "IS"=w724:dbl[], "ID"=w725:dbl[], "IG"=w723:dbl[], "error out"=w738:errorcluster, "SMU4"=w749:dbl[])  [unwired: 12 in]
        n194 = Unbundle By Name(w752) -> ("V2 Step"=w751:dbl, "V2 Start"=w750:dbl, "Number of points"=w712:i32)
        n195 = call "4155C Split array.vi"("Number of VAR2 steps"=w712, "Y2 data in"=w725, "X data in"=w746, "Y1 data in"=w724, "Y3 data in"=w723, "error in (no error)"=w738) -> ("Array of clusters"=w739:cluster{"Y data in":dbl[], "X data in":dbl[]}[], "error out"=w700:errorcluster)  [unwired: 1 in]
        n196 = case shown="True" "Plot output curve extrema vs time" {
          tunnel: w745 -> [w808 w878]
          tunnel: w736 -> [w809 w873]
          tunnel: w727 -> [w803 w869]
          tunnel: w726 -> [w802 w868]
          tunnel: w725 -> [_ w865]
          tunnel: w724 -> [_ w863]
          tunnel: w723 -> [_ w862]
          tunnel: w722 -> [w810 w858]
          tunnel: w721 -> [w811 w857]
          tunnel: w720 -> [w806 w854]
          tunnel: w719 -> [w807 w853]
          tunnel: w718 -> [w804 w850]
          tunnel: w717 -> [w805 w849]
          tunnel: w716 -> [w800 w846]
          tunnel: w715 -> [w801 w845]
          tunnel: w714 -> [_ w838]
          tunnel: [w806 w833] -> w713
          tunnel: w712 -> [_ w832]
          tunnel: [w807 w831] -> w711
          tunnel: [w808 w830] -> w710
          tunnel: [w809 w829] -> w709
          tunnel: [w810 w828] -> w708
          tunnel: [w811 w827] -> w707
          tunnel: [w800 w826] -> w706
          tunnel: [w801 w825] -> w705
          tunnel: [w802 w824] -> w704
          tunnel: [w803 w823] -> w703
          tunnel: [w804 w822] -> w702
          tunnel: [w805 w821] -> w701
          tunnel: w700 -> [w812 w820]
          tunnel: [w812 w816] -> w699
          frame False {
          }
          frame True {
            # "Adjusts graph colors."
            # "Adjusts graph colors."
            # "Ion will be the middle element of the array. The calculation of the index is done only once, since Is, Id, and Ig have the same dimensions."
            # "abs(Ig)"
            # "abs(Is)"
            # "Y1: Is\nY2: Id\nY3: Ig"
            # "abs(Id)"
            # "Adjusts graph colors."
            # "Adjusts graph colors."
            # "Adjusts graph colors."
            n197 = Absolute Value(x=w863) -> (abs(x)=w848:dbl[])
            n198 = Absolute Value(x=w865) -> (abs(x)=w864:dbl[])
            n199 = Absolute Value(x=w862) -> (abs(x)=w851:dbl[])
            n200 = Array Size(array=w864) -> (size(s)=w872:i32)
            n201 = Divide(x=w872, y=2) -> (x/y=w815:dbl)
            n202 = Subtract(x=w815, y=1) -> (x-y=w814:dbl)
            n203 = Array Max & Min(array=w848) -> (max value=w855:dbl, min value=w856:dbl)  [unwired: 2 out]
            n204 = Array Max & Min(array=w864) -> (max value=w877:dbl, min value=w861:dbl)  [unwired: 2 out]
            n205 = Array Max & Min(array=w851) -> (max value=w860:dbl, min value=w859:dbl)  [unwired: 2 out]
            n206 = Index Array(array=w848, index=w814) -> (element=w839:dbl)
            n207 = Index Array(array=w848, index=0) -> (element=w840:dbl)
            n208 = Index Array(array=w864, index=w814) -> (element=w841:dbl)
            n209 = Index Array(array=w864, index=0) -> (element=w842:dbl)
            n210 = Index Array(array=w851, index=w814) -> (element=w844:dbl)
            n211 = Index Array(array=w851, index=0) -> (element=w843:dbl)
            n212 = local write "Ig max"(w860) -> ()
            n213 = local write "Ig min"(w859) -> ()
            n214 = local write "Is max"(w855) -> ()
            n215 = local write "Is min"(w856) -> ()
            n216 = local write "Id max"(w877) -> ()
            n217 = local write "Id min"(w861) -> ()
            n218 = Build Array (concatenate)(w854, w855) -> (w833:dbl[])
            n219 = Build Array (concatenate)(w853, w856) -> (w831:dbl[])
            n220 = local write "Is off"(w840) -> ()
            n221 = local write "Is on"(w839) -> ()
            n222 = Build Array (concatenate)(w878, w877) -> (w830:dbl[])
            n223 = Build Array (concatenate)(w873, w861) -> (w829:dbl[])
            n224 = Build Array (concatenate)(w858, w860) -> (w828:dbl[])
            n225 = Build Array (concatenate)(w857, w859) -> (w827:dbl[])
            n226 = Build Array (concatenate)(w846, w839) -> (w826:dbl[])
            n227 = Build Array (concatenate)(w845, w840) -> (w825:dbl[])
            n228 = Build Array (concatenate)(w868, w841) -> (w824:dbl[])
            n229 = Build Array (concatenate)(w869, w842) -> (w823:dbl[])
            n230 = Build Array (concatenate)(w850, w844) -> (w822:dbl[])
            n231 = Build Array (concatenate)(w849, w843) -> (w821:dbl[])
            n232 = local write "Ig off"(w843) -> ()
            n233 = local write "Ig on"(w844) -> ()
            n234 = local write "Id off"(w842) -> ()
            n235 = local write "Id on"(w841) -> ()
            n236 = control-ref of="Imax vs time"() -> (w867:refnum<vi>)
            n237 = control-ref of="Imin vs time"() -> (w866:refnum<vi>)
            n238 = control-ref of="Ion vs time"() -> (w835:refnum<vi>)
            n239 = control-ref of="Ioff vs time"() -> (w834:refnum<vi>)
            n240 = control-ref of="I vs Vg"() -> (w876:refnum<vi>)
            n241 = call "4155C Split array.vi"("Number of VAR2 steps"=w832, "Y2 data in"=w824, "X data in"=w838, "Y1 data in"=w826, "Y3 data in"=w822, "error in (no error)"=w820) -> ("Array of clusters"=w836:cluster{"Y data in":dbl[], "X data in":dbl[]}[], "error out"=w819:errorcluster)  [unwired: 1 in]
            n242 = call "4155C Split array.vi"("Number of VAR2 steps"=w832, "Y2 data in"=w823, "X data in"=w838, "Y1 data in"=w825, "Y3 data in"=w821, "error in (no error)"=w819) -> ("Array of clusters"=w837:cluster{"Y data in":dbl[], "X data in":dbl[]}[], "error out"=w818:errorcluster)  [unwired: 1 in]
            n243 = call "4155C Split array.vi"("Number of VAR2 steps"=w832, "Y2 data in"=w830, "X data in"=w838, "Y1 data in"=w833, "Y3 data in"=w828, "error in (no error)"=w818) -> ("Array of clusters"=w875:cluster{"Y data in":dbl[], "X data in":dbl[]}[], "error out"=w817:errorcluster)  [unwired: 1 in]
            n244 = call "4155C Split array.vi"("Number of VAR2 steps"=w832, "Y2 data in"=w829, "X data in"=w838, "Y1 data in"=w831, "Y3 data in"=w827, "error in (no error)"=w817) -> ("Array of clusters"=w874:cluster{"Y data in":dbl[], "X data in":dbl[]}[], "error out"=w816:errorcluster)  [unwired: 1 in]
            n245 = call "4155C Config Chart Colours.vi"("Numeric"=w832, "XY Graph 2"=w867) -> ()  [unwired: 6 in]
            n246 = call "4155C Config Chart Colours.vi"("Numeric"=w832, "XY Graph 2"=w866) -> ()  [unwired: 6 in]
            n247 = call "4155C Config Chart Colours.vi"("Numeric"=w832, "XY Graph 2"=w835) -> ()  [unwired: 6 in]
            n248 = call "4155C Config Chart Colours.vi"("Numeric"=w832, "XY Graph 2"=w834) -> ()  [unwired: 6 in]
            n249 = call "4155C Config Chart Colours.vi"("Numeric"=w832, "XY Graph 2"=w876) -> ()  [unwired: 6 in]
            n250 = local write "Imax vs time"(w875) -> ()
            n251 = local write "Imin vs time"(w874) -> ()
            n252 = local write "Ion vs time"(w836) -> ()
            n253 = local write "Ioff vs time"(w837) -> ()
          }
        }
        n254 = local write "I vs Vd"(w739) -> ()
        n255 = Open/Create/Replace File(file path (use dialog)=w791, error in=w699, operation (0:open)=w747) -> (refnum out=w734:refnum<file>, error out=w732:errorcluster)  [unwired: 3 in, 1 out]
        n256 = call "4155C Make Big 2d array.vi"("1D Var1"=w746, "1d IS"=w724, "1d ID"=w725, "1d IG"=w723, "1d SMU4"=w749, "SMU4"=w694, "VAR2 START"=w750, "Number of VAR2 steps"=w712, "VAR2 STEP"=w751, "VAR1 Name"="Vd", "Decimal places in header"=i8 1, "VAR2 Name"="Vg") -> ("Header array"=w735:string[], "Data array"=w733:dbl[][])  [unwired: 14 in]
        n257 = call "4155C Write array to file.vi"("Byte Stream File Refnum"=w734, "Header"=w735, "Data Array"=w733, "error in (no error)"=w732) -> ("dup refnum"=w731:refnum<file>, "error out"=w730:errorcluster)  [unwired: 1 in]
        n258 = Close File(refnum=w731, error in=w730) -> (error out=w786:errorcluster)  [unwired: 1 out]
      }
      frame "output-fpp" {
        n259 = Number To Decimal String(number=w896) -> (decimal integer string=w950:string)  [unwired: 1 in]
        n260 = Bundle By Name(cluster=w926, "Emergency Stop"=w953) -> (w963:T1)
        n261 = Delete From Array(array=w941, index=0 ("Index")) -> (deleted portion=w939:string, array with subset deleted=w938:string[])  [unwired: 1 in]
        n262 = VISA Write(VISA resource name=w917, write buffer=":PAGE:CHAN:MODE SWE;" ("write buffer (\"\")"), error in (no error)=w914) -> (VISA resource name out=w916:refnum<visa-resource-name>, error out=w915:errorcluster)  [unwired: 1 out]
        n263 = Concatenate Strings(w949, "-outputfpp-" ("Substring"), w950, w895, ".txt" ("Substring")) -> (w952:string)
        n264 = case shown="\"d\", Default" w939 {
          tunnel: [w964 w965] -> w937
          frame "s" {
            w964 = u16 0 items=["Single", "Double"] ("sweep mode")
          }
          frame "d", Default {
            w965 = u16 1 items=["Single", "Double"] ("sweep mode")
          }
        }
        n265 = Fract/Exp String To Number(string=w938) -> (number=w920:dbl[])  [unwired: 3 in, 1 out]
        n266 = String To Path(string=w952) -> (path=w948:path)
        n267 = Index Array(array=w920, index #1=0 ("Index")) -> (element #1=w936:dbl, element #2=w935:dbl, element #3=w934:dbl)  [unwired: 2 in]
        n268 = Delete From Array(array=w920, length=3 ("Length"), index=0 ("Index")) -> (array with subset deleted=w919:dbl[])  [unwired: 1 out]
        n269 = Bundle By Name(cluster=w928, "Gate Start"=w936, "Gate Stop"=w935, "Gate Step (linear only)"=w934, "Gate Compliance"=w946, "Range mode"=w912, "Range"=w911) -> (w962:T6)
        n270 = Index Array(array=w919, index #1=0 ("Index")) -> (element #1=w931:dbl, element #2=w930:dbl, element #3=w929:dbl)  [unwired: 2 in]
        n271 = call <vilib>:"compatOverwrite.vi"("overwrite (F)"=TRUE) -> ("overwrite?"=w900:T8)
        n272 = Bundle By Name(cluster=w927, "Drain Start"=w931, "Drain Stop"=w930, "Drain Step"=w929, "Drain Compliance"=w947, "Range mode"=w910, "Range"=w913) -> (w961:T7)
        n273 = call "4155C Output-FPP.vi"("VISA resource name in"=w916, "Gate"=w962, "Drain"=w961, "Timings"=w945, "error in (no error)"=w915, "sweep mode"=w937, "Panel controls"=w963) -> ("VD"=w905:dbl[], "Outparams"=w908:T9, "VISA Resource Name out"=w943:refnum<visa-resource-name>, "Vprobe2"=w904:dbl[], "ID"=w903:dbl[], "IG"=w902:dbl[], "Vprobe1"=w901:dbl[], "error out"=w944:errorcluster)  [unwired: 13 in]
        n274 = Unbundle By Name(w908) -> ("V2 Step"=w909:dbl, "V2 Start"=w907:dbl, "Number of points"=w906:i32)
        n275 = Open/Create/Replace File(file path (use dialog)=w948, error in=w944, operation (0:open)=w900) -> (refnum out=w958:refnum<file>, error out=w959:errorcluster)  [unwired: 3 in, 1 out]
        n276 = call "4155C Make Big 2d array FPP.vi"("1D Var1"=w905, "1d ID"=w903, "1d Vp2"=w904, "1d IG"=w902, "1d Vp1"=w901, "VAR2 START"=w907, "Number of VAR2 steps"=w906, "VAR2 STEP"=w909, "VAR1 Name"="Vd", "Decimal places in header"=i8 1, "VAR2 Name"="Vg") -> ("Header array"=w954:string[], "Data array"=w955:dbl[][])  [unwired: 15 in]
        n277 = call "4155C Write array to file.vi"("Byte Stream File Refnum"=w958, "Header"=w954, "Data Array"=w955, "error in (no error)"=w959) -> ("dup refnum"=w956:refnum<file>, "error out"=w957:errorcluster)  [unwired: 1 in]
        n278 = Close File(refnum=w956, error in=w957) -> (error out=w942:errorcluster)  [unwired: 1 out]
      }
      frame "itime" {
        n279 = Delete From Array(array=w969, index=1) -> (deleted portion=w968:string)  [unwired: 1 in, 1 out]
        n280 = Delete From Array(array=w969, index=0 ("Index")) -> (deleted portion=w997:string)  [unwired: 1 in, 1 out]
        n281 = Fract/Exp String To Number(string=w968) -> (number=w967:dbl)  [unwired: 3 in, 1 out]
        n282 = case shown="\"l\"" w997 {
          tunnel: w996 -> [w1002 w1004 w1008]
          tunnel: [w1001 w1003 w1007] -> w989
          tunnel: w967 -> [w999 _ w1006]
          frame "s" {
            w1000 = u32 0 items=["short  ", "medium  ", "long  "] ("integration time 2")
            n283 = Bundle By Name(cluster=w1002, "integration time"=w1000, "Short/Long integration time"=w999) -> (w1001:T4)
          }
          frame "m", Default {
            w1005 = u32 1 items=["short  ", "medium  ", "long  "] ("integration time 2")
            n284 = Bundle By Name(cluster=w1004, "integration time"=w1005) -> (w1003:T4)
          }
          frame "l" {
            w1009 = u32 2 items=["short  ", "medium  ", "long  "] ("integration time 2")
            n285 = Bundle By Name(cluster=w1008, "integration time"=w1009, "Short/Long integration time"=w1006) -> (w1007:T4)
          }
        }
      }
      frame "pulsed" {
        n286 = Delete From Array(array=w1038, index=0 ("Index")) -> (deleted portion=w1039:string, array with subset deleted=w1026:string[])  [unwired: 1 in]
        n287 = case shown="\"on\", Default" w1039 {
          tunnel: w1037 -> [w1049 w1052]
          tunnel: [w1048 w1051] -> w1030
          tunnel: w1026 -> [w1046 _]
          frame "on", Default {
            w1047 = u16 1 items=["Continuous", "Pulsed"] ("sweep method")
            n288 = Fract/Exp String To Number(string=w1046) -> (number=w1044:dbl[])  [unwired: 3 in, 1 out]
            n289 = Index Array(array=w1044, index #1=0 ("Index")) -> (element #1=w1043:dbl, element #2=w1042:dbl, element #3=w1041:dbl)  [unwired: 2 in]
            n290 = Bundle By Name(cluster=w1049, "sweep method"=w1047, "Pulse period"=w1043, "Base voltage"=w1042, "Pulse width"=w1041) -> (w1048:T4)
          }
          frame "off" {
            w1050 = u16 0 items=["Continuous", "Pulsed"] ("sweep method")
            n291 = Bundle By Name(cluster=w1052, "sweep method"=w1050) -> (w1051:T4)
          }
        }
      }
      frame "gaterangemode" {
        n292 = Delete From Array(array=w1079, index=0 ("Index")) -> (deleted portion=w1080:string)  [unwired: 1 in, 1 out]
        n293 = case shown="\"f\"" w1080 {
          tunnel: [w1082 w1083 w1084] -> w1069
          frame "a", Default {
            w1082 = u16 0 items=["Auto", "Limited", "Fixed"] ("Gate Range\nmode 2")
          }
          frame "f" {
            w1083 = u16 2 items=["Auto", "Limited", "Fixed"] ("Gate Range\nmode 2")
          }
          frame "l" {
            w1084 = u16 1 items=["Auto", "Limited", "Fixed"] ("Gate Range\nmode 2")
          }
        }
      }
      frame "gaterange" {
        (unwired) u8 11 items=["10fA  ", "100fA  ", "1nA  ", "10nA", "100nA", "1uA", "10uA", "100uA", "1mA", "10mA", "100mA", "1A"] ("Gate Range 2")
        n294 = Delete From Array(array=w1118, index=0 ("Index")) -> (deleted portion=w1108:string)  [unwired: 1 in, 1 out]
        n295 = Scan Value(string=w1108, format string="") -> (value=w1106:dbl)  [unwired: 1 in, 1 out]
        n296 = Logarithm Base 10(1:w1106) -> (0:w1105:dbl)
        n297 = Round To Nearest(number=w1105) -> (nearest integer value=w1104:dbl)
        n298 = Add(x=w1104, y=11.0) -> (x+y=w1102:dbl)
        n299 = To Unsigned Byte Integer(number=w1102) -> (unsigned 8bit integer=w1101:u8)
      }
      frame "drainrange" {
        (unwired) u8 11 items=["10fA  ", "100fA  ", "1nA  ", "10nA", "100nA", "1uA", "10uA", "100uA", "1mA", "10mA", "100mA", "1A"] ("Gate Range 2")
        n300 = Delete From Array(array=w1153, index=0 ("Index")) -> (deleted portion=w1144:string)  [unwired: 1 in, 1 out]
        n301 = Scan Value(string=w1144, format string="") -> (value=w1142:dbl)  [unwired: 1 in, 1 out]
        n302 = Logarithm Base 10(1:w1142) -> (0:w1141:dbl)
        n303 = Round To Nearest(number=w1141) -> (nearest integer value=w1140:dbl)
        n304 = Add(x=w1140, y=11.0) -> (x+y=w1138:dbl)
        n305 = To Unsigned Byte Integer(number=w1138) -> (unsigned 8bit integer=w1137:u8)
      }
      frame "drainrangemode" {
        n306 = Delete From Array(array=w1181, index=0 ("Index")) -> (deleted portion=w1182:string)  [unwired: 1 in, 1 out]
        n307 = case shown="\"f\"" w1182 {
          tunnel: [w1184 w1185 w1186] -> w1171
          frame "a", Default {
            w1184 = u16 0 items=["Auto", "Limited", "Fixed"] ("Gate Range\nmode 2")
          }
          frame "f" {
            w1185 = u16 2 items=["Auto", "Limited", "Fixed"] ("Gate Range\nmode 2")
          }
          frame "l" {
            w1186 = u16 1 items=["Auto", "Limited", "Fixed"] ("Gate Range\nmode 2")
          }
        }
      }
      frame "Error", Default {
      }
      frame "logfile" {
        n308 = Number To Decimal String(number=w1229) -> (decimal integer string=w1264:string)  [unwired: 1 in]
        n309 = Concatenate Strings(w1263, "logfile" ("Substring"), w1264, w1227, ".txt" ("Substring")) -> (w1261:string)
        n310 = String To Path(string=w1261) -> (path=w1234:path)
        n311 = Unbundle(w1260) -> ("integration time"=w1259:u32, "Short/Long integration time"=w1258:dbl, "hold time (sec)"=w1257:dbl, "delay time (sec)"=w1256:dbl, "Step Time (0 disables)"=w1255:dbl, "sweep method"=w1254:u16, "Pulse period"=w1253:dbl, "Base voltage"=w1252:dbl, "Pulse width"=w1251:dbl)
        n312 = Build Array(w1259, w1258, w1257, w1256, w1255, w1254, w1253, w1252, w1251, w1245, w1246, w1247, w1248, w1249, w1250) -> (w1238:dbl[])
        n313 = Insert Into Array(array=dbl[][] [] ("Input Array"), new element=w1238) -> (w1237:dbl[][])  [unwired: 2 in]
        n314 = call <vilib>:"compatOverwrite.vi"("overwrite (F)"=TRUE) -> ("overwrite?"=w1232:T8)
        n315 = Open/Create/Replace File(file path (use dialog)=w1234, error in=w1236, operation (0:open)=w1232) -> (refnum out=w1242:refnum<file>, error out=w1241:errorcluster)  [unwired: 3 in, 1 out]
        n316 = call "4155C Write array to file.vi"("Byte Stream File Refnum"=w1242, "Header"=string[] ["Int Time", "Short/Long Itime", "Hold time", "Delay time", "Step time", "Sweep method", "Pulse period", "Base Voltage", "Pulse width", "Drain compliance", "Gate compliance", "Gate range mode", "Gate range", "S/D range mode", "S/D range"], "Data Array"=w1237, "error in (no error)"=w1241) -> ("dup refnum"=w1244:refnum<file>, "error out"=w1243:errorcluster)  [unwired: 1 in]
        n317 = Close File(refnum=w1244, error in=w1243) -> (error out=w1235:errorcluster)  [unwired: 1 out]
      }
      frame "sample" {
        w1268 = 1
        # "Add a time offset (elapsed time) to the time axis."
        # "Adjusts graph colors."
        n318 = Number To Decimal String(number=w1306) -> (decimal integer string=w1348:string)  [unwired: 1 in]
        n319 = Fract/Exp String To Number(string=w1345) -> (number=w1310:dbl[])  [unwired: 3 in, 1 out]
        n320 = Concatenate Strings(w1326, "-sample-" ("Substring"), w1348, w1304, ".txt" ("Substring")) -> (w1346:string)
        n321 = Index Array(array=w1310, index=0 ("Index")) -> (element=w1343:dbl)
        n322 = String To Path(string=w1346) -> (path=w1330:path)
        n323 = Index Array(array=w1310, index=2 ("Index")) -> (element=w1339:dbl)
        n324 = Index Array(array=w1310, index=3 ("Index")) -> (element=w1312:dbl)
        n325 = Index Array(array=w1310, index=4 ("Index")) -> (element=w1309:dbl)
        n326 = call "4155C Config Sampling Measurements.vi"("Sampling interval"=w1309, "Sample time"=w1312, "Display on/off"=TRUE, "Timings"=w1318, "Num Points"=w1339, "error in (no error)"=w1350, "Drain Compliance"=w1349, "Gate Compliance"=w1327, "VISA session"=w1351) -> ("error out"=w1352:errorcluster, "dup VISA resource name"=w1353:refnum<visa-resource-name>)  [unwired: 1 in]
        n327 = Index Array(array=w1310, index=1 ("Index")) -> (element=w1340:dbl)
        n328 = local read "Plot sample extrema vs time"() -> (w1274:bool)
        n329 = call "4155C Take Sample.vi"("Emergency Stop"=w1323, "error in (no error)"=w1352, "Vd"=w1340, "Vg"=w1343, "VISA resource name in"=w1353) -> ("error out"=w1271:errorcluster, "Id"=w1279:dbl[], "Ig"=w1280:dbl[], "VISA Resource Name out"=w1320:refnum<visa-resource-name>, "Is"=w1281:dbl[], "Time"=w1267:dbl[])  [unwired: 1 in]
        n330 = Add(x=w1267, y=w1266) -> (x+y=w1272:dbl[])
        n331 = case shown="True" w1274 {
          tunnel: w1275 -> [w1354 w1356]
          tunnel: [w1354 w1357] -> w1273
          tunnel: w1272 -> [_ w1355]
          frame False {
          }
          frame True {
            n332 = Insert Into Array(array=w1356, new element=w1355) -> (w1357:i32[])  [unwired: 1 in]
          }
        }
        n333 = case shown="True" "Plot sample extrema vs time" {
          tunnel: w1281 -> [_ w1385]
          tunnel: w1279 -> [_ w1386]
          tunnel: w1280 -> [_ w1387]
          tunnel: [w1364 w1374] -> w1270
          tunnel: w1271 -> [w1364 w1378]
          tunnel: w1299 -> [w1363 w1390]
          tunnel: w1298 -> [w1362 w1389]
          tunnel: w1297 -> [w1361 w1391]
          tunnel: w1296 -> [w1360 w1388]
          tunnel: w1295 -> [w1359 w1393]
          tunnel: w1294 -> [w1358 w1392]
          tunnel: [w1363 w1376] -> w1293
          tunnel: [w1362 w1369] -> w1292
          tunnel: [w1361 w1370] -> w1291
          tunnel: [w1360 w1394] -> w1290
          tunnel: [w1359 w1377] -> w1289
          tunnel: [w1358 w1371] -> w1288
          tunnel: w1273 -> [_ w1365]
          frame False {
          }
          frame True {
            w1372 = 1
            # "Number of VAR2 steps is 1."
            # "abs(Ig)"
            # "abs(Is)"
            # "abs(Id)"
            # "Adjusts graph colors."
            n334 = Absolute Value(x=w1387) -> (abs(x)=w1366:dbl[])
            n335 = Absolute Value(x=w1386) -> (abs(x)=w1367:dbl[])
            n336 = Absolute Value(x=w1385) -> (abs(x)=w1368:dbl[])
            n337 = Array Max & Min(array=w1368) -> (max value=w1384:dbl, min value=w1381:dbl)  [unwired: 2 out]
            n338 = Array Max & Min(array=w1367) -> (max value=w1383:dbl, min value=w1380:dbl)  [unwired: 2 out]
            n339 = Array Max & Min(array=w1366) -> (max value=w1382:dbl, min value=w1379:dbl)  [unwired: 2 out]
            n340 = local write "Id max"(w1383) -> ()
            n341 = local write "Id min"(w1380) -> ()
            n342 = local write "Ig max"(w1382) -> ()
            n343 = local write "Ig min"(w1379) -> ()
            n344 = Insert Into Array(array=w1393, new element=w1366) -> (w1377:dbl[])  [unwired: 1 in]
            n345 = Insert Into Array(array=w1392, new element=w1366) -> (w1371:dbl[])  [unwired: 1 in]
            n346 = local write "Is max"(w1384) -> ()
            n347 = local write "Is min"(w1381) -> ()
            n348 = Insert Into Array(array=w1391, new element=w1367) -> (w1370:dbl[])  [unwired: 1 in]
            n349 = Insert Into Array(array=w1388, new element=w1367) -> (w1394:dbl[])  [unwired: 1 in]
            n350 = Insert Into Array(array=w1390, new element=w1368) -> (w1376:dbl[])  [unwired: 1 in]
            n351 = Insert Into Array(array=w1389, new element=w1368) -> (w1369:dbl[])  [unwired: 1 in]
            n352 = control-ref of="Imax vs time"() -> (w1395:refnum<vi>)
            n353 = call "4155C Config Chart Colours.vi"("Numeric"=w1372, "XY Graph 2"=w1395) -> ()  [unwired: 6 in]
            n354 = call "4155C Split array.vi"("Number of VAR2 steps"=w1372, "Y2 data in"=w1370, "X data in"=w1365, "Y1 data in"=w1376, "Y3 data in"=w1377, "error in (no error)"=w1378) -> ("Array of clusters"=w1396:cluster{"Y data in":dbl[], "X data in":dbl[]}[], "error out"=w1375:errorcluster)  [unwired: 1 in]
            n355 = call "4155C Split array.vi"("Number of VAR2 steps"=w1372, "Y2 data in"=w1370, "X data in"=w1365, "Y1 data in"=w1369, "Y3 data in"=w1371, "error in (no error)"=w1375) -> ("Array of clusters"=w1373:cluster{"Y data in":dbl[], "X data in":dbl[]}[], "error out"=w1374:errorcluster)  [unwired: 1 in]
            n356 = local write "Imax vs time"(w1396) -> ()
            n357 = local write "Imin vs time"(w1373) -> ()
          }
        }
        n358 = control-ref of="I vs time (Bias Stress)"() -> (w1278:refnum<vi>)
        n359 = Insert Into Array(array=dbl[][] [] ("Input Array"), new element=w1272) -> (w1276:dbl[][])  [unwired: 2 in]
        n360 = call "4155C Split array.vi"("Number of VAR2 steps"=w1268, "Y2 data in"=w1279, "X data in"=w1272, "Y1 data in"=w1281, "Y3 data in"=w1280, "error in (no error)"=w1270) -> ("Array of clusters"=w1277:cluster{"Y data in":dbl[], "X data in":dbl[]}[], "error out"=w1269:errorcluster)  [unwired: 1 in]
        n361 = Insert Into Array(array=w1276, new element=w1280) -> (w1333:dbl[][])  [unwired: 2 in]
        n362 = VISA Write(VISA resource name=w1320, write buffer=":DISP ON" ("write buffer (\"\")"), error in (no error)=w1269) -> (VISA resource name out=w1319:refnum<visa-resource-name>, error out=w1321:errorcluster)  [unwired: 1 out]
        n363 = Insert Into Array(array=w1333, new element=w1279) -> (w1332:dbl[][])  [unwired: 2 in]
        n364 = call "4155C Config Chart Colours.vi"("Numeric"=w1268, "XY Graph 2"=w1278) -> ()  [unwired: 6 in]
        n365 = local write "I vs time (Bias Stress)"(w1277) -> ()
        n366 = Insert Into Array(array=w1332, new element=w1281) -> (w1325:dbl[][])  [unwired: 2 in]
        n367 = Transpose 2D Array(2D array=w1325) -> (transposed array=w1324:dbl[][])
        n368 = call <vilib>:"compatOverwrite.vi"("overwrite (F)"=TRUE) -> ("overwrite?"=w1307:T8)
        n369 = Open/Create/Replace File(file path (use dialog)=w1330, error in=w1321, operation (0:open)=w1307) -> (refnum out=w1336:refnum<file>, error out=w1335:errorcluster)  [unwired: 3 in, 1 out]
        n370 = call "4155C Write array to file.vi"("Byte Stream File Refnum"=w1336, "Header"=string[] ["Time /s", "Ig /A", "Id /A", "Is /A"], "Data Array"=w1324, "error in (no error)"=w1335) -> ("dup refnum"=w1338:refnum<file>, "error out"=w1337:errorcluster)  [unwired: 1 in]
        n371 = Close File(refnum=w1338, error in=w1337) -> (error out=w1328:errorcluster)  [unwired: 1 out]
      }
      frame "samplei" {
        n372 = Number To Decimal String(number=w1413) -> (decimal integer string=w1464:string)  [unwired: 1 in]
        n373 = Concatenate Strings(w1443, "-samplei-" ("Substring"), w1464, w1412, ".txt" ("Substring")) -> (w1462:string)
        n374 = Fract/Exp String To Number(string=w1461) -> (number=w1428:dbl[])  [unwired: 3 in, 1 out]
        n375 = String To Path(string=w1462) -> (path=w1446:path)
        n376 = Index Array(array=w1428, index=4 ("Index")) -> (element=w1422:dbl)
        n377 = Index Array(array=w1428, index=3 ("Index")) -> (element=w1423:dbl)
        n378 = Index Array(array=w1428, index=1 ("Index")) -> (element=w1425:dbl)
        n379 = Index Array(array=w1428, index=0 ("Index")) -> (element=w1426:dbl)
        n380 = Index Array(array=w1428, index=2 ("Index")) -> (element=w1424:dbl)
        n381 = call "4155C Config SamplingI Measurements.vi"("Sample time"=w1424, "Display on/off"=TRUE, "Timings"=w1435, "Num Points"=w1425, "error in (no error)"=w1466, "Sampling interval"=w1423, "VISA session"=w1467) -> ("error out"=w1468:errorcluster, "dup VISA resource name"=w1469:refnum<visa-resource-name>)  [unwired: 3 in]
        n382 = call "4155C Take SampleI.vi"("Emergency Stop"=w1440, "error in (no error)"=w1468, "Idg 2"=w1426, "Vdg compliance 2"=w1422, "VISA resource name in"=w1469) -> ("error out"=w1438:errorcluster, "Idg"=w1471:dbl[], "Vdg"=w1448:dbl[], "VISA Resource Name out"=w1436:refnum<visa-resource-name>, "Is"=w1470:dbl[], "Time"=w1452:dbl[])  [unwired: 1 in]
        n383 = Insert Into Array(array=dbl[][] [] ("Input Array"), new element=w1452) -> (w1451:dbl[][])  [unwired: 2 in]
        n384 = Insert Into Array(array=w1451, new element=w1448) -> (w1450:dbl[][])  [unwired: 2 in]
        n385 = Insert Into Array(array=w1450, new element=w1471) -> (w1449:dbl[][])  [unwired: 2 in]
        n386 = VISA Write(VISA resource name=w1436, write buffer=":DISP ON" ("write buffer (\"\")"), error in (no error)=w1438) -> (VISA resource name out=w1421:refnum<visa-resource-name>, error out=w1437:errorcluster)  [unwired: 1 out]
        n387 = Insert Into Array(array=w1449, new element=w1470) -> (w1442:dbl[][])  [unwired: 2 in]
        n388 = call <vilib>:"compatOverwrite.vi"("overwrite (F)"=TRUE) -> ("overwrite?"=w1416:T8)
        n389 = Open/Create/Replace File(file path (use dialog)=w1446, error in=w1437, operation (0:open)=w1416) -> (refnum out=w1455:refnum<file>, error out=w1454:errorcluster)  [unwired: 3 in, 1 out]
        n390 = Transpose 2D Array(2D array=w1442) -> (transposed array=w1441:dbl[][])
        n391 = call "4155C Write array to file.vi"("Byte Stream File Refnum"=w1455, "Header"=string[] ["Time /s", "Vdg /V", "Idg /A", "Is /A"], "Data Array"=w1441, "error in (no error)"=w1454) -> ("dup refnum"=w1457:refnum<file>, "error out"=w1456:errorcluster)  [unwired: 1 in]
        n392 = Close File(refnum=w1457, error in=w1456) -> (error out=w1419:errorcluster)  [unwired: 1 out]
        n393 = VISA Write(VISA resource name=w1421, write buffer=";:PAGE:SCON:STAN OFF;:PAGE:CHAN:VSU2:DIS;" ("write buffer (\"\")"), error in (no error)=w1419) -> (VISA resource name out=w1417:refnum<visa-resource-name>, error out=w1418:errorcluster)  [unwired: 1 out]
      }
      frame "#" {
        n394 = VISA Write(VISA resource name=w1492, write buffer=":DISP ON" ("write buffer (\"\")"), error in (no error)=w1491) -> (VISA resource name out=w1490:refnum<visa-resource-name>, error out=w1489:errorcluster)  [unwired: 1 out]
      }
      frame "stressV" {
        n395 = Number To Decimal String(number=w1516) -> (decimal integer string=w1557:string)  [unwired: 1 in]
        n396 = Concatenate Strings(w1541, "-stressV-" ("Substring"), w1557, w1515, ".txt" ("Substring")) -> (w1555:string)
        n397 = Fract/Exp String To Number(string=w1554) -> (number=w1527:dbl[])  [unwired: 3 in, 1 out]
        n398 = String To Path(string=w1555) -> (path=w1545:path)
        n399 = Index Array(array=w1527, index=3 ("Index")) -> (element=w1524:dbl)
        n400 = Index Array(array=w1527, index=1 ("Index")) -> (element=w1522:dbl)
        n401 = Index Array(array=w1527, index=0 ("Index")) -> (element=w1521:dbl)
        n402 = Index Array(array=w1527, index=4 ("Index")) -> (element=w1526:dbl)
        n403 = Index Array(array=w1527, index=2 ("Index")) -> (element=w1523:dbl)
        n404 = call "4155C Config V Stress.vi"("VISA session"=w1560, "ID compliance"=w1524, "VD"=w1522, "VG"=w1521, "IG compliance"=w1523, "error in (no error)"=w1559, "Display on/off"=TRUE) -> ("dup VISA resource name"=w1562:refnum<visa-resource-name>, "error out"=w1561:errorcluster)
        n405 = call "4155C Apply Stress.vi"("error in (no error)"=w1561, "Duration"=w1526, "Emergency Stop"=w1540, "VISA resource name in"=w1562) -> ("error out"=w1538:errorcluster, "VISA Resource Name out"=w1536:refnum<visa-resource-name>)
        n406 = VISA Write(VISA resource name=w1536, write buffer=":DISP ON" ("write buffer (\"\")"), error in (no error)=w1538) -> (VISA resource name out=w1535:refnum<visa-resource-name>, error out=w1537:errorcluster)  [unwired: 1 out]
        n407 = call <vilib>:"compatOverwrite.vi"("overwrite (F)"=TRUE) -> ("overwrite?"=w1520:T8)
        n408 = Open/Create/Replace File(file path (use dialog)=w1545, error in=w1537, operation (0:open)=w1520) -> (refnum out=w1548:refnum<file>, error out=w1547:errorcluster)  [unwired: 3 in, 1 out]
        n409 = call "4155C Write array to file.vi"("Byte Stream File Refnum"=w1548, "Header"=string[] ["V stress completed successfully", ""], "error in (no error)"=w1547) -> ("dup refnum"=w1550:refnum<file>, "error out"=w1549:errorcluster)  [unwired: 2 in]
        n410 = Close File(refnum=w1550, error in=w1549) -> (error out=w1543:errorcluster)  [unwired: 1 out]
      }
      frame "stressI" {
        n411 = Number To Decimal String(number=w1578) -> (decimal integer string=w1615:string)  [unwired: 1 in]
        n412 = Concatenate Strings(w1599, "-stressI-" ("Substring"), w1615, w1577, ".txt" ("Substring")) -> (w1613:string)
        n413 = Fract/Exp String To Number(string=w1612) -> (number=w1587:dbl[])  [unwired: 3 in, 1 out]
        n414 = Index Array(array=w1587, index=1 ("Index")) -> (element=w1583:dbl)
        n415 = Index Array(array=w1587, index=0 ("Index")) -> (element=w1584:dbl)
        n416 = call "4155C Config I Stress.vi"("VISA session"=w1618, "IDG"=w1584, "VDG compliance"=w1583, "error in (no error)"=w1617, "Display on/off"=TRUE) -> ("dup VISA resource name"=w1620:refnum<visa-resource-name>, "error out"=w1619:errorcluster)
        n417 = Index Array(array=w1587, index=2 ("Index")) -> (element=w1585:dbl)
        n418 = String To Path(string=w1613) -> (path=w1603:path)
        n419 = call "4155C Apply Stress.vi"("error in (no error)"=w1619, "Duration"=w1585, "Emergency Stop"=w1598, "VISA resource name in"=w1620) -> ("error out"=w1596:errorcluster, "VISA Resource Name out"=w1594:refnum<visa-resource-name>)
        n420 = VISA Write(VISA resource name=w1594, write buffer=":DISP ON" ("write buffer (\"\")"), error in (no error)=w1596) -> (VISA resource name out=w1593:refnum<visa-resource-name>, error out=w1595:errorcluster)  [unwired: 1 out]
        n421 = call <vilib>:"compatOverwrite.vi"("overwrite (F)"=TRUE) -> ("overwrite?"=w1582:T8)
        n422 = Open/Create/Replace File(file path (use dialog)=w1603, error in=w1595, operation (0:open)=w1582) -> (refnum out=w1606:refnum<file>, error out=w1605:errorcluster)  [unwired: 3 in, 1 out]
        n423 = call "4155C Write array to file.vi"("Byte Stream File Refnum"=w1606, "Header"=string[] ["I stress completed successfully", ""], "error in (no error)"=w1605) -> ("dup refnum"=w1608:refnum<file>, "error out"=w1607:errorcluster)  [unwired: 2 in]
        n424 = Close File(refnum=w1608, error in=w1607) -> (error out=w1601:errorcluster)  [unwired: 1 out]
      }
      frame "vsu2pulse" {
        n425 = Number To Decimal String(number=w1636) -> (decimal integer string=w1671:string)  [unwired: 1 in]
        n426 = Concatenate Strings(w1656, "-vsu2-" ("Substring"), w1671, w1635, ".txt" ("Substring")) -> (w1669:string)
        n427 = Fract/Exp String To Number(string=w1668) -> (number=w1644:dbl[])  [unwired: 3 in, 1 out]
        n428 = String To Path(string=w1669) -> (path=w1660:path)
        n429 = Index Array(array=w1644, index=1 ("Index")) -> (element=w1643:dbl)
        n430 = Index Array(array=w1644, index=0 ("Index")) -> (element=w1641:dbl)
        n431 = call "4155C Config VSU2 Stress.vi"("error in (no error)"=w1673, "VSU2"=w1641, "Display on/off"=TRUE, "VISA session"=w1674) -> ("error out"=w1675:errorcluster, "dup VISA resource name"=w1676:refnum<visa-resource-name>)
        n432 = call "4155C Apply Stress.vi"("error in (no error)"=w1675, "Duration"=w1643, "Emergency Stop"=w1655, "VISA resource name in"=w1676) -> ("error out"=w1653:errorcluster, "VISA Resource Name out"=w1651:refnum<visa-resource-name>)
        n433 = VISA Write(VISA resource name=w1651, write buffer=":DISP ON" ("write buffer (\"\")"), error in (no error)=w1653) -> (VISA resource name out=w1650:refnum<visa-resource-name>, error out=w1652:errorcluster)  [unwired: 1 out]
        n434 = call <vilib>:"compatOverwrite.vi"("overwrite (F)"=TRUE) -> ("overwrite?"=w1640:T8)
        n435 = Open/Create/Replace File(file path (use dialog)=w1660, error in=w1652, operation (0:open)=w1640) -> (refnum out=w1663:refnum<file>, error out=w1662:errorcluster)  [unwired: 3 in, 1 out]
        n436 = call "4155C Write array to file.vi"("Byte Stream File Refnum"=w1663, "Header"=string[] ["VSU2 pulse completed successfully", ""], "error in (no error)"=w1662) -> ("dup refnum"=w1665:refnum<file>, "error out"=w1664:errorcluster)  [unwired: 2 in]
        n437 = Close File(refnum=w1665, error in=w1664) -> (error out=w1658:errorcluster)  [unwired: 1 out]
      }
      frame "sample-fpp" {
        w1703 = string[] ["Time /s", "Id VgVd /A", "Ig VgVd /A", "Vp1 VgVd /V", "Vp2 VgVd /V"] ("Header")
        w1707 = "%d" ("format string")
        n438 = Number To Decimal String(number=w1692) -> (decimal integer string=w1755:string)  [unwired: 1 in]
        n439 = Fract/Exp String To Number(string=w1752) -> (number=w1740:dbl[])  [unwired: 3 in, 1 out]
        n440 = Concatenate Strings(w1746, "-samplefpp-" ("Substring"), w1755, w1691, ".txt" ("Substring")) -> (w1753:string)
        n441 = String To Path(string=w1753) -> (path=w1715:path)
        n442 = Index Array(array=w1740, index=0 ("Index")) -> (element=w1701:dbl)
        n443 = Index Array(array=w1740, index=1 ("Index")) -> (element=w1700:dbl)
        n444 = Index Array(array=w1740, index=2 ("Index")) -> (element=w1748:dbl)
        n445 = Index Array(array=w1740, index=3 ("Index")) -> (element=w1738:dbl)
        n446 = call "4155C Config Sampling Measurements FPP.vi"("VISA session"=w1758, "Num Points"=w1748, "Vg"=w1701, "Display on/off"=TRUE, "Gate Compliance"=w1747, "Drain Compliance"=w1756, "Standby"="Standby", "error in (no error)"=w1757, "Timings"=w1745, "Vd"=w1700, "Sample time"=w1738) -> ("dup VISA resource name"=w1717:refnum<visa-resource-name>, "error out"=w1716:errorcluster)  [unwired: 3 in]
        n447 = Number To Decimal String(number=w1701) -> (decimal integer string=w1727:string)  [unwired: 1 in]
        n448 = call "4155C Take Sample FPP.vi"("VISA resource name in"=w1717, "error in (no error)"=w1716, "Emergency Stop"=w1718) -> ("Time"=w1722:dbl[], "Vp1"=w1732:dbl[], "VISA Resource Name out"=w1698:refnum<visa-resource-name>, "Ig"=w1720:dbl[], "Id"=w1721:dbl[], "Vp2"=w1730:dbl[], "error out"=w1719:errorcluster)  [unwired: 10 in]
        n449 = Insert Into Array(array=dbl[][] [] ("Input Array"), new element=w1722) -> (w1736:dbl[][])  [unwired: 2 in]
        n450 = Number To Decimal String(number=w1700) -> (decimal integer string=w1725:string)  [unwired: 1 in]
        n451 = Insert Into Array(array=w1736, new element=w1721) -> (w1735:dbl[][])  [unwired: 2 in]
        n452 = Concatenate Strings("(Vg = " ("Substring"), w1727, "V, Vd = " ("Substring"), w1725, "V)" ("Substring")) -> (w1723:string)
        n453 = Insert Into Array(array=w1735, new element=w1720) -> (w1734:dbl[][])  [unwired: 2 in]
        n454 = Insert Into Array(array=w1734, new element=w1732) -> (w1731:dbl[][])  [unwired: 2 in]
        n455 = Insert Into Array(array=w1731, new element=w1730) -> (w1699:dbl[][])  [unwired: 2 in]
        n456 = Transpose 2D Array(2D array=w1699) -> (transposed array=w1729:dbl[][])
        n457 = call <vilib>:"compatOverwrite.vi"("overwrite (F)"=TRUE) -> ("overwrite?"=w1696:T8)
        n458 = Open/Create/Replace File(file path (use dialog)=w1715, error in=w1719, operation (0:open)=w1696) -> (refnum out=w1712:refnum<file>, error out=w1713:errorcluster)  [unwired: 3 in, 1 out]
        n459 = Array To Spreadsheet String(array=w1703, 3:w1707) -> (spreadsheet string=w1709:string)  [unwired: 1 in]
        n460 = Search and Replace String(replace all?=TRUE ("replace all? (F)"), input string=w1709, search string="VgVd", replace string=w1723) -> (result string=w1705:string)  [unwired: 4 in, 3 out]
        n461 = Spreadsheet String To Array(format string=w1707, spreadsheet string=w1705, array type (2D Dbl)=w1703) -> (array=w1704:string[])  [unwired: 1 in]
        n462 = call "4155C Write array to file.vi"("Byte Stream File Refnum"=w1712, "Header"=w1704, "Data Array"=w1729, "error in (no error)"=w1713) -> ("dup refnum"=w1710:refnum<file>, "error out"=w1711:errorcluster)  [unwired: 1 in]
        n463 = Close File(refnum=w1710, error in=w1711) -> (error out=w1697:errorcluster)  [unwired: 1 out]
      }
      frame "resample-fpp" {
        w1787 = string[] ["Time /s", "Id VgVd /A", "Ig VgVd /A", "Vp1 VgVd /V", "Vp2 VgVd /V"] ("Header")
        w1791 = "%d" ("format string")
        n464 = Number To Decimal String(number=w1773) -> (decimal integer string=w1831:string)  [unwired: 1 in]
        n465 = Fract/Exp String To Number(string=w1828) -> (number=w1780:dbl[])  [unwired: 3 in, 1 out]
        n466 = Concatenate Strings(w1824, "-resamplefpp-" ("Substring"), w1831, w1774, ".txt" ("Substring")) -> (w1829:string)
        n467 = String To Path(string=w1829) -> (path=w1799:path)
        n468 = Index Array(array=w1780, index=0 ("Index")) -> (element=w1786:dbl)
        n469 = Index Array(array=w1780, index=1 ("Index")) -> (element=w1785:dbl)
        n470 = Number To Decimal String(number=w1786) -> (decimal integer string=w1809:string)  [unwired: 1 in]
        n471 = call "4155C Take Sample FPP.vi"("VISA resource name in"=w1782, "error in (no error)"=w1781, "Emergency Stop"=w1800) -> ("Time"=w1804:dbl[], "Vp1"=w1814:dbl[], "VISA Resource Name out"=w1784:refnum<visa-resource-name>, "Ig"=w1802:dbl[], "Id"=w1803:dbl[], "Vp2"=w1812:dbl[], "error out"=w1801:errorcluster)  [unwired: 10 in]
        n472 = Insert Into Array(array=dbl[][] [] ("Input Array"), new element=w1804) -> (w1818:dbl[][])  [unwired: 2 in]
        n473 = Number To Decimal String(number=w1785) -> (decimal integer string=w1807:string)  [unwired: 1 in]
        n474 = Insert Into Array(array=w1818, new element=w1803) -> (w1817:dbl[][])  [unwired: 2 in]
        n475 = Concatenate Strings("(Vg = " ("Substring"), w1809, "V, Vd = " ("Substring"), w1807, "V)" ("Substring")) -> (w1805:string)
        n476 = Insert Into Array(array=w1817, new element=w1802) -> (w1816:dbl[][])  [unwired: 2 in]
        n477 = Insert Into Array(array=w1816, new element=w1814) -> (w1813:dbl[][])  [unwired: 2 in]
        n478 = Insert Into Array(array=w1813, new element=w1812) -> (w1779:dbl[][])  [unwired: 2 in]
        n479 = call <vilib>:"compatOverwrite.vi"("overwrite (F)"=TRUE) -> ("overwrite?"=w1778:T8)
        n480 = Open/Create/Replace File(file path (use dialog)=w1799, error in=w1801, operation (0:open)=w1778) -> (refnum out=w1796:refnum<file>, error out=w1797:errorcluster)  [unwired: 3 in, 1 out]
        n481 = Array To Spreadsheet String(array=w1787, 3:w1791) -> (spreadsheet string=w1793:string)  [unwired: 1 in]
        n482 = Transpose 2D Array(2D array=w1779) -> (transposed array=w1811:dbl[][])
        n483 = Search and Replace String(replace all?=TRUE ("replace all? (F)"), input string=w1793, search string="VgVd", replace string=w1805) -> (result string=w1789:string)  [unwired: 4 in, 3 out]
        n484 = Spreadsheet String To Array(format string=w1791, spreadsheet string=w1789, array type (2D Dbl)=w1787) -> (array=w1788:string[])  [unwired: 1 in]
        n485 = call "4155C Write array to file.vi"("Byte Stream File Refnum"=w1796, "Header"=w1788, "Data Array"=w1811, "error in (no error)"=w1797) -> ("dup refnum"=w1794:refnum<file>, "error out"=w1795:errorcluster)  [unwired: 1 in]
        n486 = Close File(refnum=w1794, error in=w1795) -> (error out=w1783:errorcluster)  [unwired: 1 out]
      }
      frame "serial" {
        n487 = local read "Termination char\n(0xA = '\\n' = LF)\n(0xD = '\\r' = CR)"() -> (w1854:u8)
        n488 = local read "Enable Termination\nChar (T)"() -> (w1855:bool)
        n489 = Index Array(array=w1862, index=0 ("Index")) -> (element=w1861:string)
        n490 = local read "parity"() -> (w1845:u16)
        n491 = local read "Delay before read (ms)"() -> (w1856:u32)
        n492 = local read "byte count"() -> (w1853:u32)
        n493 = local read "Timeout (ms)"() -> (w1852:u32)
        n494 = local read "VISA resource name"() -> (w1849:refnum<visa-resource-name>)
        n495 = local read "baud rate"() -> (w1848:u32)
        n496 = local read "Serial End Mode for Reads"() -> (w1847:u16)
        n497 = local read "data bits"() -> (w1846:u16)
        n498 = local read "stop bits"() -> (w1851:u16)
        n499 = local read "flow control"() -> (w1850:u16)
        n500 = call "Serial write and read v0.5.vi"("Delay before read (ms)"=w1856, "Termination char\n(0xA = '\\n' = LF)\n(0xD = '\\r' = CR)"=w1854, "Enable Termination\nChar (T)"=w1855, "parity"=w1845, "stop bits"=w1851, "string to write"=w1861, "flow control"=w1850, "byte count"=w1853, "Serial Settings:Serial End Mode for Reads"=w1847, "Timeout (ms)"=w1852, "error in (no error)"=w1867, "VISA resource name"=w1849, "baud rate"=w1848, "data bits"=w1846) -> ("Serial port output"=w1857:string, "error out"=w1866:errorcluster)
        n501 = Build Array (concatenate)(w1857, w1858) -> (w1859:string[])
      }
    }
    n502 = local read "Time Units"() -> (w68:u16)
    n503 = case shown="0" w68 {
      tunnel: ["Time (Seconds)" ("element") "Time (Minutes)" ("element") "Time (Hours)" ("element")] -> w108
      frame 0 {
      }
      frame 1, Default {
      }
      frame 2 {
      }
    }
    n504 = Build Array(w120, w76, w86, w85, w84, w83, w82, w81, w80, w79, w78, w77, w75) -> (w141:dbl[][])
    n505 = Transpose 2D Array(2D array=w141) -> (transposed array=w140:dbl[][])
    n506 = Concatenate Strings(w73, "-Imax_Imin_Ion_Ioff_vs_time.txt" ("Suffix (Imax,Imin,Ion,Ioff)")) -> (w151:string)
    n507 = Build Array(w108, "Is max (A)" ("VAR2 Name"), "Is min (A)" ("VAR2 Name"), "Id max (A)" ("VAR2 Name"), "Id min (A)" ("VAR2 Name"), "Ig max (A)" ("VAR2 Name"), "Ig min (A)" ("VAR2 Name"), "Is on (A)" ("VAR2 Name"), "Is off (A)" ("VAR2 Name"), "Id on (A)" ("VAR2 Name"), "Id off (A)" ("VAR2 Name"), "Ig on (A)" ("VAR2 Name"), "Ig off (A)" ("VAR2 Name")) -> (w146:string[])
    n508 = Array To Spreadsheet String(array=w140, 3:"%e" ("format string")) -> (spreadsheet string=w144:string)  [unwired: 1 in]
    n509 = Array To Spreadsheet String(array=w146, 3:"" ("format string")) -> (spreadsheet string=w145:string)  [unwired: 1 in]
    n510 = String To Path(string=w151) -> (path=w150:path)
    n511 = Build Array(w145, w144) -> (w143:string[])
    n512 = Write to Text File(file (use dialog)=w150, text=w143, error in=w119) -> (refnum out=w152:refnum<file>, error out=w142:errorcluster)  [unwired: 1 in, 1 out]
    n513 = Close File(refnum=w152, error in=w142) -> (error out=w72:errorcluster)  [unwired: 1 out]
    n514 = Concatenate Strings(w73, "-serial_port_output.txt" ("Suffix (serial port log)")) -> (w122:string)
    n515 = String To Path(string=w122) -> (path=w121:path)
    n516 = Build Array(w108, "Serial port input" ("VAR2 Name"), "Serial port output: ") -> (w112:string[])
    n517 = Array To Spreadsheet String(array=w116, 3:"" ("format string")) -> (spreadsheet string=w109:string)  [unwired: 1 in]
    n518 = Array To Spreadsheet String(array=w112, 3:"" ("format string")) -> (spreadsheet string=w110:string)  [unwired: 1 in]
    n519 = Build Array(w110, w109) -> (w111:string[])
    n520 = Array To Spreadsheet String(array=w115, 3:"" ("format string")) -> (spreadsheet string=w127:string)  [unwired: 1 in]
    n521 = Write to Text File(file (use dialog)=w121, text=w111, error in=w72) -> (refnum out=w123:refnum<file>, error out=w124:errorcluster)  [unwired: 1 in, 1 out]
    n522 = Close File(refnum=w123, error in=w124) -> (error out=w70:errorcluster)  [unwired: 1 out]
    n523 = local write "Serial port data"(w127) -> ()
  }
  "error out" <- w27
  "Timings Indicator" <- w18
  "SMU4 Indicator" <- w2
  "Is max" <- w12
  "Id max" <- w12
  "Ig max" <- w12
  "Imax vs time" <- w1
  "I vs Vg" <- w1
  "Imin vs time" <- w1
  "I vs Vd" <- w1
  "Serial port data" <- "" ("Serial port data")
  "Is min" <- w11
  "Id min" <- w11
  "Ig min" <- w11
  "Ion vs time" <- w1
  "Ioff vs time" <- w1
  "Is on" <- w10
  "Id on" <- w10
  "Ig on" <- w10
  "Is off" <- w9
  "Id off" <- w9
  "Ig off" <- w9
  "I vs time (Bias Stress)" <- w1
